vi "Auto.vi"() -> ()   [LabVIEW 2020]
uses:
  Global_Variable/A180648.vi
  Global_Variable/Global.vi
  Global_Variable/System_Conf.vi
  <userlib>/_MGI/1D Array/MGI Running Average/MGI Running Average(DBL).vi
  <userlib>/_MGI/1D Array/MGI Running Average/MGI Running Average(SGL).vi
  Libraries/S7/S7.lvlib
panel:
  out "磨合正向初始化":bool
  out "磨合逆向初始化":bool
  out "试验项_Event":refnum<user-event>
  out "产品变更_Event":refnum<user-event>
  out "NVH":bool=TRUE
  out "T1+T2":dbl
  out "T2":dbl
  out "T1":dbl
  out "吸收电流":sgl
  out "输出扭矩(大)":sgl
  out "输入扭矩":sgl
  out "力特性逆向去程":bool
  out "力特性正向去程":bool
  out "力特性逆向回程":bool
  out "力特性正向回程":bool
  out "逆向空载正向初始化":bool
  out "逆向空载逆向初始化":bool
  out "功能正向初始化":bool
  out "功能逆向初始化":bool
  out "空载逆向初始化":bool
  out "空载正向初始化":bool
  out "布尔":bool=TRUE
  out "当前车速":i32
  out "试验项目":T1(tab)
  out "空载试验":cluster{dbl[], dbl[]}[](graph)
  out "功能试验":cluster{dbl[], dbl[]}[](graph)
  out "力特性试验":cluster{dbl[], dbl[]}[](graph)
  out "电流特性试验":cluster{dbl[], dbl[]}[](graph)
  out "传感器特性试验":cluster{dbl[], dbl[]}[](graph)
  out "逆向空载试验":cluster{dbl[], dbl[]}[](graph)
  out "磨合":cluster{dbl[], dbl[]}[](graph)
  out "振动2NHV-FFT":cluster{"f0":dbl, "df":dbl, "magnitude":dbl[]}[](graph)
  out "振动1NVH-FFT":cluster{"f0":dbl, "df":dbl, "magnitude":dbl[]}[](graph)
  in  "判定结果":bool[][](array[boolean])=[[TRUE]]
  in  "STEP":string
  # "车速0"
  # "车速1"
  # "车速2"
  # "车速3"
  # "车速4"
  # "车速5"
  # "车速0"
  # "车速1"
  # "车速2"
  # "车速3"
  # "车速4"
  # "车速5"
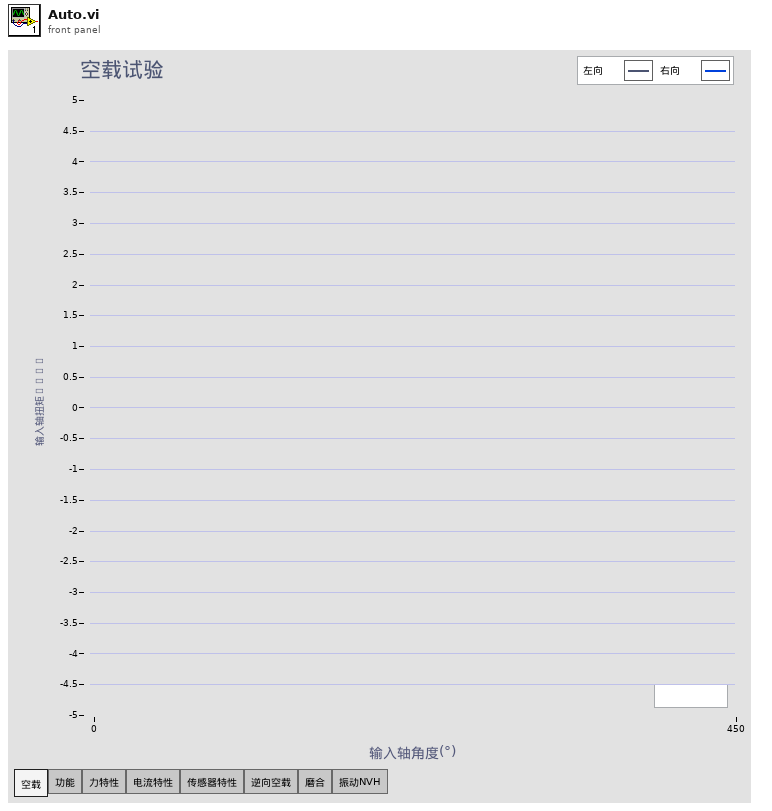
[diagram p1: front panel]
types:
  T1 = enum32{"空载", "功能", "力特性", "电流特性", "传感器特性", "逆向空载", "磨合", "振动NVH"}
  T2 = enum32{"Invalid", "Standard", "Closed", "Hidden", "Minimized", "Maximized"}
  T3 = enum32{"空载", "功能", "力特性", "电流特性", "传感器特性", "逆向空载", "振动NVH", "磨合", "完成"}
  T4 = enum16{"Left Button", "Center Button", "Right Button", "Window Close"}
  T5 = enum16{"角度标定状态", "角度标定", "角度标定清除", "扭矩标定状态", "扭矩标定", "扭矩标定清除", "内部软件版本号", "客户软件版本号"}
  T6 = enum16{"客户软件版本号", "角度标定状态", "角度标定", "角度标定清除", "扭矩标定状态", "扭矩标定", "扭矩标定清除", "内部软件版本号"}
  T7 = cluster{"输入轴扭矩":dbl, "输出轴扭矩小量程":dbl, "输出轴扭矩大量程":dbl}
  T8 = typedef "System_conf.ctl" = cluster{"空载滤波":bool, "逆向空载滤波":bool, "空载扭矩系数":dbl, "逆向空载扭矩系数":dbl}
  T9 = cluster{"扭矩判定范围":cluster{"单位":string, "下限":dbl, "上限":dbl}, "正向扭矩最大值":cluster{"单位":string, "下限":dbl, "上限":dbl}, "正向扭矩最小值":cluster{"单位":string, "下限":dbl, "上限":dbl}, "正向扭矩平均值":cluster{"单位":string, "下限":dbl, "上限":dbl}, "正向扭矩波动值":cluster{"单位":string, "下限":dbl, "上限":dbl}, "逆向扭矩最大值":cluster{"单位":string, "下限":dbl, "上限":dbl}, "逆向扭矩最小值":cluster{"单位":string, "下限":dbl, "上限":dbl}, "逆向扭矩平均值":cluster{"单位":string, "下限":dbl, "上限":dbl}, "逆向扭矩波动值":cluster{"单位":string, "下限":dbl, "上限":dbl}, "正逆向扭矩差值":cluster{"单位":string, "下限":dbl, "上限":dbl}, "启动力矩":cluster{"单位":string, "下限":dbl, "上限":dbl}}
  T10 = cluster{"扭矩判定范围":cluster{"单位":string, "下限":dbl, "上限":dbl}, "正向扭矩最大值":cluster{"单位":string, "下限":dbl, "上限":dbl}, "正向扭矩最小值":cluster{"单位":string, "下限":dbl, "上限":dbl}, "正向扭矩平均值":cluster{"单位":string, "下限":dbl, "上限":dbl}, "正向扭矩波动值":cluster{"单位":string, "下限":dbl, "上限":dbl}, "逆向扭矩最大值":cluster{"单位":string, "下限":dbl, "上限":dbl}, "逆向扭矩最小值":cluster{"单位":string, "下限":dbl, "上限":dbl}, "逆向扭矩平均值":cluster{"单位":string, "下限":dbl, "上限":dbl}, "逆向扭矩波动值":cluster{"单位":string, "下限":dbl, "上限":dbl}, "正逆向扭矩差值":cluster{"单位":string, "下限":dbl, "上限":dbl}}
  T11 = cluster{"对称性检测点":cluster{"单位":string, "下限":dbl, "上限":dbl}, "对称度":cluster{"单位":string, "下限":dbl, "上限":dbl}, "目标输出扭矩1":cluster{"单位":string, "下限":dbl, "上限":dbl}, "目标1正向输入扭矩":cluster{"单位":string, "下限":dbl, "上限":dbl}, "目标1逆向输入扭矩":cluster{"单位":string, "下限":dbl, "上限":dbl}, "目标1正逆向扭矩差":cluster{"单位":string, "下限":dbl, "上限":dbl}, "目标1输入扭矩滞后":cluster{"单位":string, "下限":dbl, "上限":dbl}, "目标输出扭矩2":cluster{"单位":string, "下限":dbl, "上限":dbl}, "目标2正向输入扭矩":cluster{"单位":string, "下限":dbl, "上限":dbl}, "目标2逆向输入扭矩":cluster{"单位":string, "下限":dbl, "上限":dbl}, "目标2正逆向扭矩差":cluster{"单位":string, "下限":dbl, "上限":dbl}, "目标2输入扭矩滞后":cluster{"单位":string, "下限":dbl, "上限":dbl}, "目标输出扭矩3":cluster{"单位":string, "下限":dbl, "上限":dbl}, "目标3正向输入扭矩":cluster{"单位":string, "下限":dbl, "上限":dbl}, "目标3逆向输入扭矩":cluster{"单位":string, "下限":dbl, "上限":dbl}, "目标3正逆向扭矩差":cluster{"单位":string, "下限":dbl, "上限":dbl}, "目标3输入扭矩滞后":cluster{"单位":string, "下限":dbl, "上限":dbl}, "目标输出扭矩4":cluster{"单位":string, "下限":dbl, "上限":dbl}, "目标4正向输入扭矩":cluster{"单位":string, "下限":dbl, "上限":dbl}, "目标4逆向输入扭矩":cluster{"单位":string, "下限":dbl, "上限":dbl}, "目标4正逆向扭矩差":cluster{"单位":string, "下限":dbl, "上限":dbl}, "目标4输入扭矩滞后":cluster{"单位":string, "下限":dbl, "上限":dbl}, "目标输出扭矩5":cluster{"单位":string, "下限":dbl, "上限":dbl}, "目标5正向输入扭矩":cluster{"单位":string, "下限":dbl, "上限":dbl}, "目标5逆向输入扭矩":cluster{"单位":string, "下限":dbl, "上限":dbl}, "目标5正逆向扭矩差":cluster{"单位":string, "下限":dbl, "上限":dbl}, "目标5输入扭矩滞后":cluster{"单位":string, "下限":dbl, "上限":dbl}}[]
  T12 = cluster{"主副信号和MAX":cluster{"单位":string, "下限":dbl, "上限":dbl}, "主副信号和MIN":cluster{"单位":string, "下限":dbl, "上限":dbl}, "主信号线性误差":cluster{"单位":string, "下限":dbl, "上限":dbl}, "副信号线性误差":cluster{"单位":string, "下限":dbl, "上限":dbl}, "主信号MAX":cluster{"单位":string, "下限":dbl, "上限":dbl}, "主信号MIN":cluster{"单位":string, "下限":dbl, "上限":dbl}, "副信号MAX":cluster{"单位":string, "下限":dbl, "上限":dbl}, "副信号MIN":cluster{"单位":string, "下限":dbl, "上限":dbl}, "中心偏移量":cluster{"单位":string, "下限":dbl, "上限":dbl}, "定点设置":cluster{"单位":string, "下限":dbl, "上限":dbl}, "定点左侧主信号":cluster{"单位":string, "下限":dbl, "上限":dbl}, "定点左侧副信号":cluster{"单位":string, "下限":dbl, "上限":dbl}, "定点右侧主信号":cluster{"单位":string, "下限":dbl, "上限":dbl}, "定点右侧副信号":cluster{"单位":string, "下限":dbl, "上限":dbl}}
  T13 = cluster{"对称性检测点":cluster{"单位":string, "下限":dbl, "上限":dbl}, "对称度":cluster{"单位":string, "下限":dbl, "上限":dbl}, "最大电流":cluster{"单位":string, "下限":dbl, "上限":dbl}, "目标输出电流1":cluster{"单位":string, "下限":dbl, "上限":dbl}, "目标1正向输入扭矩":cluster{"单位":string, "下限":dbl, "上限":dbl}, "目标1逆向输入扭矩":cluster{"单位":string, "下限":dbl, "上限":dbl}, "目标1正逆向扭矩差":cluster{"单位":string, "下限":dbl, "上限":dbl}, "目标1输入扭矩滞后":cluster{"单位":string, "下限":dbl, "上限":dbl}, "目标输出电流2":cluster{"单位":string, "下限":dbl, "上限":dbl}, "目标2正向输入扭矩":cluster{"单位":string, "下限":dbl, "上限":dbl}, "目标2逆向输入扭矩":cluster{"单位":string, "下限":dbl, "上限":dbl}, "目标2正逆向扭矩差":cluster{"单位":string, "下限":dbl, "上限":dbl}, "目标2输入扭矩滞后":cluster{"单位":string, "下限":dbl, "上限":dbl}, "目标输出电流3":cluster{"单位":string, "下限":dbl, "上限":dbl}, "目标3正向输入扭矩":cluster{"单位":string, "下限":dbl, "上限":dbl}, "目标3逆向输入扭矩":cluster{"单位":string, "下限":dbl, "上限":dbl}, "目标3正逆向扭矩差":cluster{"单位":string, "下限":dbl, "上限":dbl}, "目标3输入扭矩滞后":cluster{"单位":string, "下限":dbl, "上限":dbl}, "目标输出电流4":cluster{"单位":string, "下限":dbl, "上限":dbl}, "目标4正向输入扭矩":cluster{"单位":string, "下限":dbl, "上限":dbl}, "目标4逆向输入扭矩":cluster{"单位":string, "下限":dbl, "上限":dbl}, "目标4正逆向扭矩差":cluster{"单位":string, "下限":dbl, "上限":dbl}, "目标4输入扭矩滞后":cluster{"单位":string, "下限":dbl, "上限":dbl}, "目标输出电流5":cluster{"单位":string, "下限":dbl, "上限":dbl}, "目标5正向输入扭矩":cluster{"单位":string, "下限":dbl, "上限":dbl}, "目标5逆向输入扭矩":cluster{"单位":string, "下限":dbl, "上限":dbl}, "目标5正逆向扭矩差":cluster{"单位":string, "下限":dbl, "上限":dbl}, "目标5输入扭矩滞后":cluster{"单位":string, "下限":dbl, "上限":dbl}}[]
  T14 = cluster{"振动1频率检测段1范围":cluster{"单位":string, "下限":dbl, "上限":dbl}, "振动1频率检测段2范围":cluster{"单位":string, "下限":dbl, "上限":dbl}, "振动1频率检测段3范围":cluster{"单位":string, "下限":dbl, "上限":dbl}, "振动1频率检测段4范围":cluster{"单位":string, "下限":dbl, "上限":dbl}, "振动1频率检测段5范围":cluster{"单位":string, "下限":dbl, "上限":dbl}, "振动2频率检测段1范围":cluster{"单位":string, "下限":dbl, "上限":dbl}, "振动2频率检测段2范围":cluster{"单位":string, "下限":dbl, "上限":dbl}, "振动2频率检测段3范围":cluster{"单位":string, "下限":dbl, "上限":dbl}, "振动2频率检测段4范围":cluster{"单位":string, "下限":dbl, "上限":dbl}, "振动2频率检测段5范围":cluster{"单位":string, "下限":dbl, "上限":dbl}}
  T15 = cluster{"振动1频率检测段1振幅":cluster{"单位":string, "下限":dbl, "上限":dbl}, "振动1频率检测段2振幅":cluster{"单位":string, "下限":dbl, "上限":dbl}, "振动1频率检测段3振幅":cluster{"单位":string, "下限":dbl, "上限":dbl}, "振动1频率检测段4振幅":cluster{"单位":string, "下限":dbl, "上限":dbl}, "振动1频率检测段5振幅":cluster{"单位":string, "下限":dbl, "上限":dbl}, "振动2频率检测段1振幅":cluster{"单位":string, "下限":dbl, "上限":dbl}, "振动2频率检测段2振幅":cluster{"单位":string, "下限":dbl, "上限":dbl}, "振动2频率检测段3振幅":cluster{"单位":string, "下限":dbl, "上限":dbl}, "振动2频率检测段4振幅":cluster{"单位":string, "下限":dbl, "上限":dbl}, "振动2频率检测段5振幅":cluster{"单位":string, "下限":dbl, "上限":dbl}}
  T16 = cluster{"扭矩判定范围":cluster{"单位":string, "下限":dbl, "上限":dbl}, "正向扭矩最大值":cluster{"单位":string, "下限":dbl, "上限":dbl}, "正向扭矩最小值":cluster{"单位":string, "下限":dbl, "上限":dbl}, "正向扭矩平均值":cluster{"单位":string, "下限":dbl, "上限":dbl}, "正向扭矩波动值":cluster{"单位":string, "下限":dbl, "上限":dbl}, "逆向扭矩最大值":cluster{"单位":string, "下限":dbl, "上限":dbl}, "逆向扭矩最小值":cluster{"单位":string, "下限":dbl, "上限":dbl}, "逆向扭矩平均值":cluster{"单位":string, "下限":dbl, "上限":dbl}, "逆向扭矩波动值":cluster{"单位":string, "下限":dbl, "上限":dbl}, "正逆向扭矩差值":cluster{"单位":string, "下限":dbl, "上限":dbl}, "启动扭矩范围":cluster{"单位":string, "下限":dbl, "上限":dbl}, "启动扭矩":cluster{"单位":string, "下限":dbl, "上限":dbl}}
  T17 = cluster{"试验速度":dbl, "试验角度":dbl, "负载扭矩":dbl, "保护扭矩":dbl}
  T18 = cluster{"输入旋转位移":sgl, "输入移载位移":sgl, "工装移载位移":sgl, "输入编码位移":sgl, "输入扭矩":sgl, "输出扭矩(小)":sgl, "输出扭矩(大)":sgl, "吸收电流":sgl}
  T19 = typedef "svc_Spectrum Info.ctl" = cluster{"channel name":string, "description":string, "x-axis units":T20, "spectral info":cluster{"spectrum type":T21, "linear/dB":enum16{"linear", "dB"}, "window":u16, "window size":i32, "FFT size":i32}, "engineering units":T22, "custom label":string, "dB reference [EU]":dbl, "peak units":enum16{"rms", "peak", "peak-peak"}, "weighting filter":T23, "spectral density?":bool, "unit label":string, "spectrum skewed?":bool, "complimentary spectrum units":T24}
  T20 = typedef "svc_X-Axis Units.ctl" = u16
  T21 = typedef "svc_Spectrum Type.ctl" = enum16{"FFT Spectrum [complex]", "Amplitude [Magnitude]", "Power [Magnitude^2]", "Cross Spectrum [complex]", "Frequency Response [Complex]"}
  T22 = typedef "svc_Engineering Units Text Ring.ctl" = u16
  T23 = typedef "svc_Weighting Filter Text Ring.ctl" = u16
  T24 = typedef "svc_Complimentary Spectrum Units.ctl" = enum16{"none", "radians", "degrees", "cycles", "imaginary"}
  T25 = cluster{"启用助力":dbl, "试验速度":dbl, "试验角度":dbl, "保护扭矩":dbl}
  T26 = typedef "lveventtype.ctl" = enum32{"Null", "Timeout", "Annotation Menu Selection", "Annotation Menu Selection?", "App Instance Close", "App Instance Close?", "Autoscale Range Change", "Bookmark Info Change", "Cell Edit", "Cell Edit?", "Cursor Grab", "Cursor Grab?", "Cursor Menu Selection", "Cursor Menu Selection?", "Cursor Move", "Cursor Release", "Data Change", "Direction Change", "Display State Change", "Drag Ended", "Drag Enter", "Drag Leave", "Drag Over", "Drag Source Update", "Drag Starting", "Drag Starting?", "Drop", "Exec State Change", "Key Down", "Key Down?", "Key Repeat", "Key Repeat?", "Key Up", "Listbox Double Click", "Menu Activation?", "Menu Selection (App)", "Menu Selection? (App)", "Menu Selection (User)", "Mouse Down", "Mouse Down?", "Mouse Enter", "Mouse Leave", "Mouse Move", "Mouse Up", "Mouse Wheel", "NI Security User Change (App)", "Pane Size", "Panel Close", "Panel Close?", "Panel Resize", "Plot Attribute Change", "Scale Range Change", "Shortcut Menu Activation?", "Shortcut Menu Selection (App)", "Shortcut Menu Selection? (App)", "Shortcut Menu Selection (User)", "Tree Double Click", "Tree Drag", "Tree Drag?", "Tree Drop", "Tree Drop?", "Tree Item Close", "Tree Item Close?", "Tree Item Open", "Tree Item Open?", "User Event", "Value Change"}
  T27 = typedef "LVPoint32TypeDef.ctl" = cluster{"Horizontal":i32, "Vertical":i32}
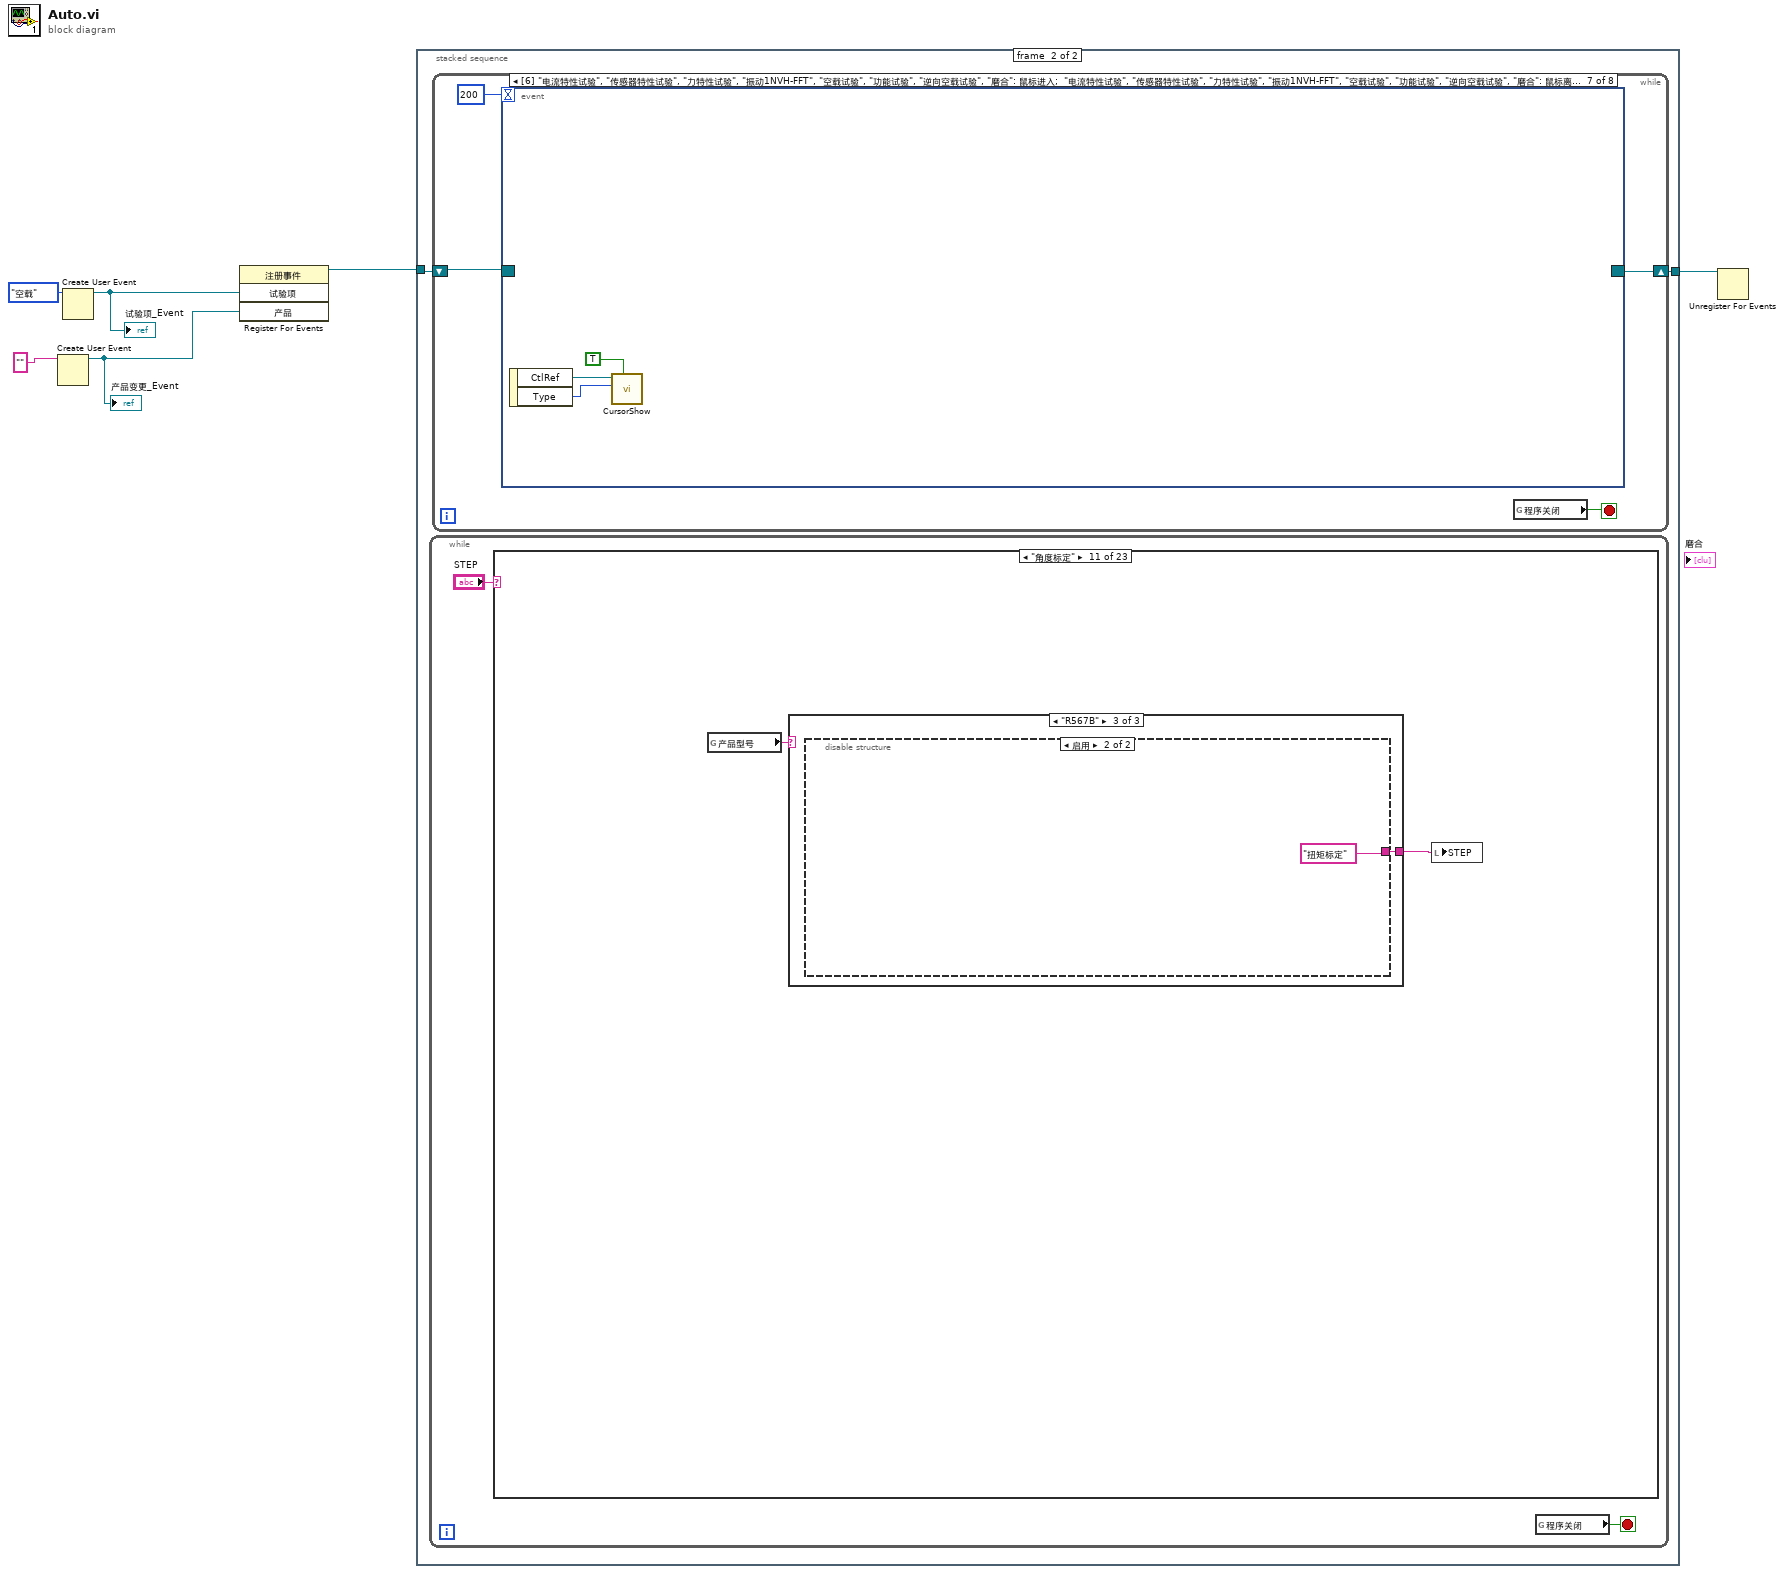
[diagram p0: block diagram]
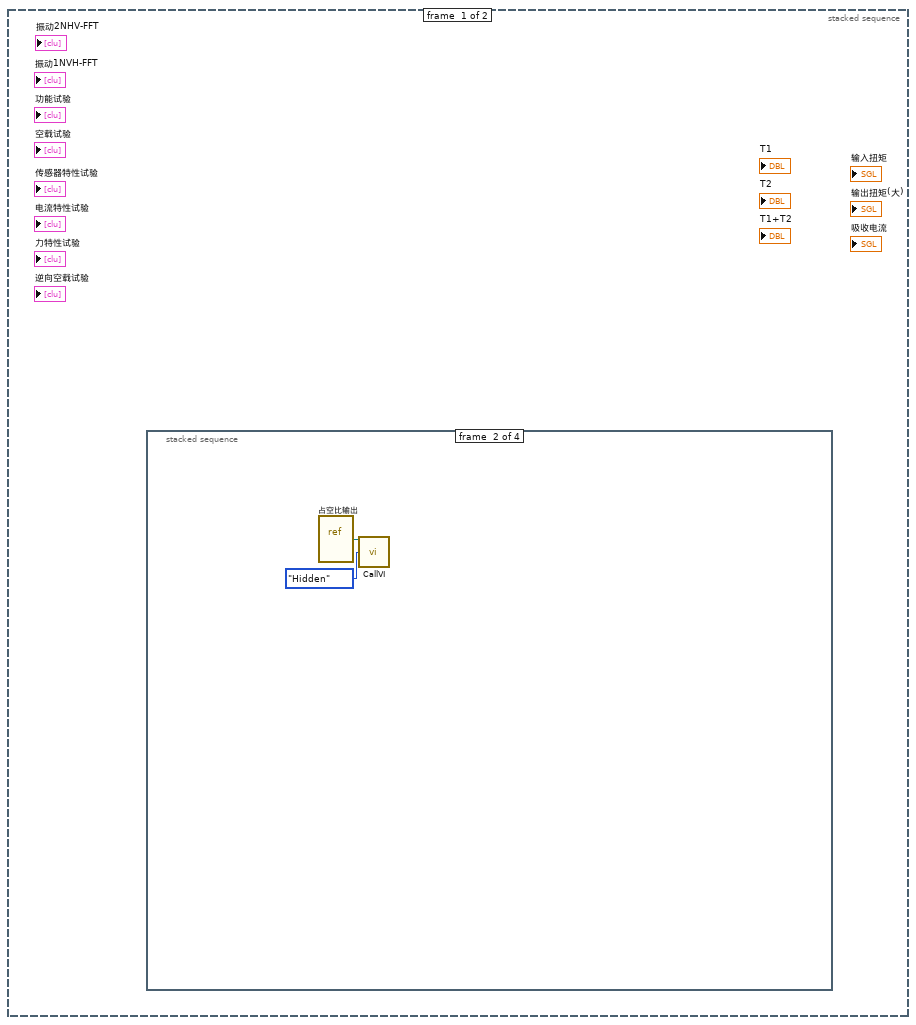
[diagram p2: hidden frame]
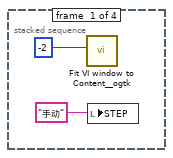
[diagram p3: hidden frame]
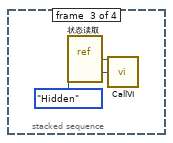
[diagram p4: hidden frame]
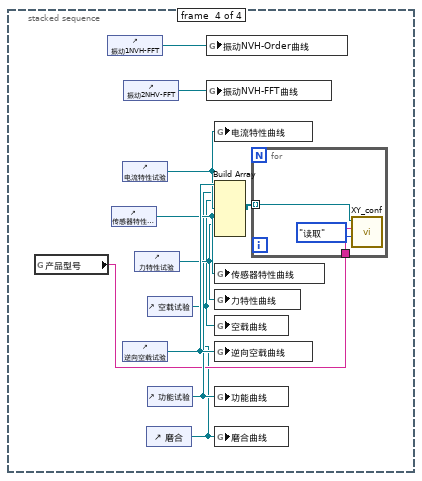
[diagram p5: hidden frame]
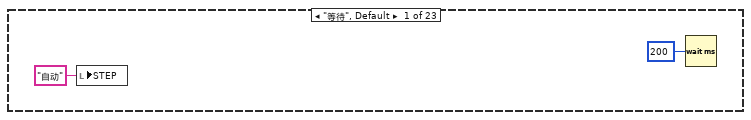
[diagram p6: hidden frame]
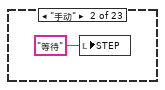
[diagram p7: hidden frame]
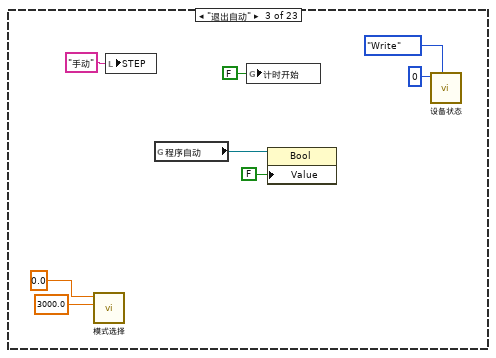
[diagram p8: hidden frame]
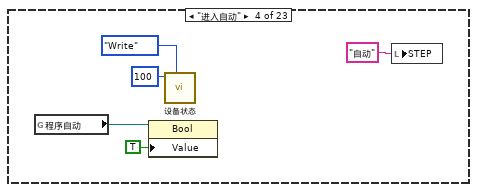
[diagram p9: hidden frame]
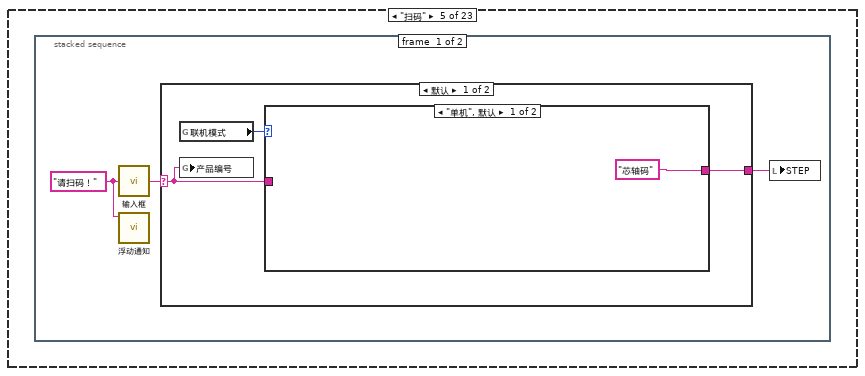
[diagram p10: hidden frame]
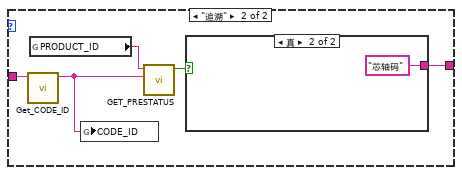
[diagram p11: hidden frame]
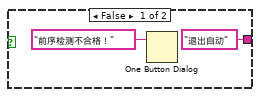
[diagram p12: hidden frame]
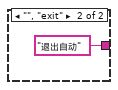
[diagram p13: hidden frame]
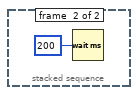
[diagram p14: hidden frame]
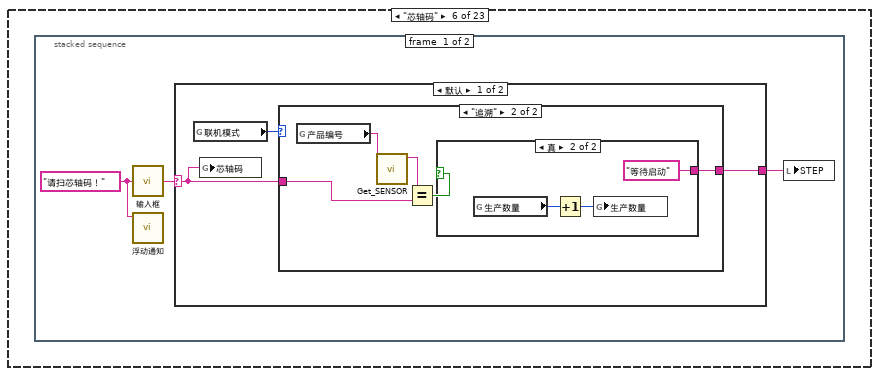
[diagram p15: hidden frame]
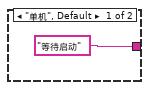
[diagram p16: hidden frame]
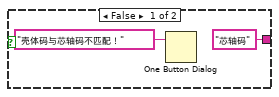
[diagram p17: hidden frame]
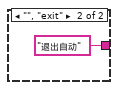
[diagram p18: hidden frame]
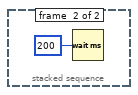
[diagram p19: hidden frame]
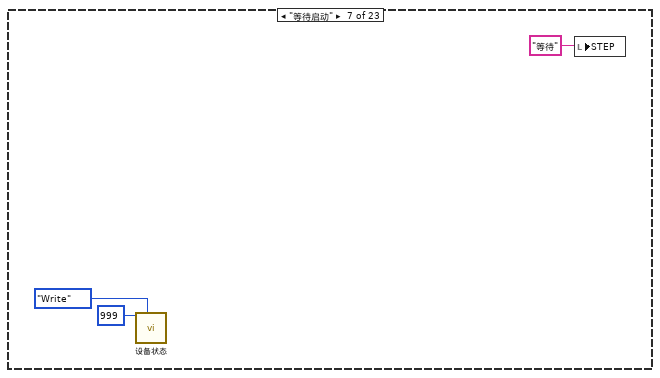
[diagram p20: hidden frame]
diagram:
  n1 = Create User Event(user event datatype="" ("产品")) -> (user event=w1:refnum<user-event>)  [unwired: 1 in, 1 out]
  "产品变更_Event" <- w1
  n2 = Create User Event(user event datatype=T1."空载" ("试验项")) -> (user event=w4:refnum<user-event>)  [unwired: 1 in, 1 out]
  "试验项_Event" <- w4
  n3 = register-events(w4, w1) -> (reference out=w5:refnum<event-registration>)  [unwired: 2 in, 1 out]
  n4 = stacked-sequence {
    tunnel: w5 -> [_ w28]
    tunnel: [_ w27] -> w3
    frame #0 {
      n5 = stacked-sequence {
        frame #0 {
          n6 = call <userlib>:"Fit VI window to Content__ogtk.vi"("border spacing (2 px)"=-2) -> ()  [unwired: 5 in, 2 out]
          n7 = local write "STEP"("手动" ("STEP")) -> ()
        }
        frame #1 {
          n8 = vi-ref "占空比输出.vi"() -> (w10:refnum<vi>)
          n9 = call "CallVI.vi"("VI引用"=w10, "状态"=T2."Hidden") -> ()  [unwired: 12 in, 2 out]
        }
        frame #2 {
          n10 = vi-ref "状态读取.vi"() -> (w12:refnum<vi>)
          n11 = call "CallVI.vi"("VI引用"=w12, "状态"=T2."Hidden") -> ()  [unwired: 12 in, 2 out]
        }
        frame #3 {
          n12 = global read "Global.vi" "产品型号"() -> (w14:string)
          n13 = control-ref of="振动1NVH-FFT"() -> (w22:refnum<vi>)
          n14 = control-ref of="传感器特性试验"() -> (w19:refnum<vi>)
          n15 = control-ref of="电流特性试验"() -> (w20:refnum<vi>)
          n16 = control-ref of="逆向空载试验"() -> (w21:refnum<vi>)
          n17 = control-ref of="振动2NHV-FFT"() -> (w23:refnum<vi>)
          n18 = control-ref of="力特性试验"() -> (w18:refnum<vi>)
          n19 = control-ref of="磨合"() -> (w13:refnum<vi>)
          n20 = control-ref of="空载试验"() -> (w16:refnum<vi>)
          n21 = control-ref of="功能试验"() -> (w17:refnum<vi>)
          n22 = global write "A180648.vi" "振动NVH-Order曲线"(w22) -> ()
          n23 = global write "A180648.vi" "振动NVH-FFT曲线"(w23) -> ()
          n24 = global write "A180648.vi" "电流特性曲线"(w20) -> ()
          n25 = Build Array(w21, w17, w16, w20, w19, w18, w13) -> (w15:refnum<vi>[])
          n26 = global write "A180648.vi" "传感器特性曲线"(w19) -> ()
          n27 = global write "A180648.vi" "力特性曲线"(w18) -> ()
          n28 = global write "A180648.vi" "空载曲线"(w16) -> ()
          n29 = global write "A180648.vi" "逆向空载曲线"(w21) -> ()
          n30 = global write "A180648.vi" "功能曲线"(w17) -> ()
          n31 = global write "A180648.vi" "磨合曲线"(w13) -> ()
          n32 = for {
            tunnel: w15 -> [w25] mode=indexing
            tunnel: w14 -> [w24]
            n33 = call "XY_conf.vi"("方式"=enum16{"写入", "读取"}."读取", "产品"=w24, "XY图引用"=w25) -> ()  [unwired: 4 in, 1 out]
          }
        }
      }
    }
    frame #1 {
      n34 = while {
        stop <- w30 stop-if-true
        n35 = case shown="\"角度标定\"" "STEP" {
          frame "等待", Default {
            n36 = local write "STEP"("自动" ("STEP")) -> ()
            n37 = Wait (ms)(milliseconds to wait=u32 200 ("等待时间（毫秒）")) -> ()  [unwired: 1 out]
          }
          frame "手动" {
            n38 = local write "STEP"("等待" ("STEP")) -> ()
          }
          frame "退出自动" {
            n39 = call-poly "模式选择.vi"("Max Torque"=sgl 3000.0, "Velocity"=sgl 0.0) -> ()  [unwired: 9 in, 1 out]
            n40 = local write "STEP"("手动" ("STEP")) -> ()
            n41 = global read "Global.vi" "程序自动"() -> (w37:refnum<vi>)
            n42 = global write "Global.vi" "计时开始"(FALSE ("计时开始")) -> ()
            n43 = property class="Bool"(reference=w37, "Value"=FALSE) -> ()  [unwired: 1 in, 2 out]
            n44 = call "设备状态.vi"("枚举"=enum16{"Read", "Write"}."Write", "Status_Write"=i16 0) -> ()  [unwired: 9 in, 1 out]
          }
          frame "进入自动" {
            n45 = global read "Global.vi" "程序自动"() -> (w43:refnum<vi>)
            n46 = property class="Bool"(reference=w43, "Value"=TRUE) -> ()  [unwired: 1 in, 2 out]
            n47 = call "设备状态.vi"("枚举"=enum16{"Read", "Write"}."Write", "Status_Write"=i16 100) -> ()  [unwired: 9 in, 1 out]
            n48 = local write "STEP"("自动" ("STEP")) -> ()
          }
          frame "扫码" {
            n49 = stacked-sequence {
              frame #0 {
                w48 = "请扫码！" ("提示信息")
                n50 = call "输入框.vi"("提示信息"=w48) -> ("条形码输出"=w49:string)
                n51 = call "浮动通知.vi"("通知内容"=w48) -> ()  [unwired: 11 in]
                n52 = case shown="默认" w49 {
                  selector: w49 -> [w51 _]
                  tunnel: [w52 "退出自动" ("State(s) in Front (\"\")")] -> w47
                  frame Default {
                    n53 = global read "Global.vi" "联机模式"() -> (w50:enum16{"单机", "追溯"})
                    n54 = global write "Global.vi" "产品编号"(w51) -> ()
                    n55 = case shown="\"单机\", 默认" w50 {
                      tunnel: ["芯轴码" ("State(s) in Front (\"\")") w58] -> w52
                      tunnel: w51 -> [_ w55]
                      frame "单机", Default {
                      }
                      frame "追溯" {
                        n56 = call "Get_CODE_ID.vi"("CODE_MAIN"=w55) -> ("CODE_ID"=w54:string)  [unwired: 10 in]
                        n57 = global read "追溯Global.vi" "PRODUCT_ID"() -> (w57:string)
                        n58 = global write "追溯Global.vi" "CODE_ID"(w54) -> ()
                        n59 = call "GET_PRESTATUS.vi"("CODE_ID"=w54, "PRODUCT_ID"=w57) -> ("OK?"=w56:bool)  [unwired: 9 in]
                        n60 = case shown="真" w56 {
                          tunnel: ["退出自动" ("State(s) in Front (\"\")") "芯轴码" ("State(s) in Front (\"\")")] -> w58
                          frame False {
                            n61 = One Button Dialog(message="前序检测不合格！" ("消息")) -> ()  [unwired: 1 in, 1 out]
                          }
                          frame True {
                          }
                        }
                      }
                    }
                  }
                  frame "", "exit" {
                  }
                }
                n62 = local write "STEP"(w47) -> ()
              }
              frame #1 {
                n63 = Wait (ms)(milliseconds to wait=u32 200 ("等待时间（毫秒）")) -> ()  [unwired: 1 out]
              }
            }
          }
          frame "芯轴码" {
            n64 = stacked-sequence {
              frame #0 {
                w65 = "请扫芯轴码！" ("提示信息")
                n65 = call "输入框.vi"("提示信息"=w65) -> ("条形码输出"=w66:string)
                n66 = call "浮动通知.vi"("通知内容"=w65) -> ()  [unwired: 11 in]
                n67 = case shown="默认" w66 {
                  selector: w66 -> [w68 _]
                  tunnel: [w69 "退出自动" ("State(s) in Front (\"\")")] -> w64
                  frame Default {
                    n68 = global read "Global.vi" "联机模式"() -> (w67:enum16{"单机", "追溯"})
                    n69 = global write "Global.vi" "芯轴码"(w68) -> ()
                    n70 = case shown="\"追溯\"" w67 {
                      tunnel: ["等待启动" ("State(s) in Front (\"\")") w75] -> w69
                      tunnel: w68 -> [_ w72]
                      frame "单机", Default {
                      }
                      frame "追溯" {
                        n71 = global read "Global.vi" "产品编号"() -> (w74:string)
                        n72 = call "Get_SENSOR.vi"("CODE_MAIN"=w74) -> ("CODE_SENSOR"=w73:string)  [unwired: 10 in]
                        n73 = Equal?(x=w73, y=w72) -> (x = y?=w71:bool)
                        n74 = case shown="真" w71 {
                          tunnel: ["芯轴码" ("State(s) in Front (\"\")") "等待启动" ("State(s) in Front (\"\")")] -> w75
                          frame False {
                            n75 = One Button Dialog(message="壳体码与芯轴码不匹配！" ("消息")) -> ()  [unwired: 1 in, 1 out]
                          }
                          frame True {
                            n76 = global read "Global.vi" "生产数量"() -> (w78:i32)
                            n77 = Increment(x=w78) -> (x+1=w79:i32)
                            n78 = global write "Global.vi" "生产数量"(w79) -> ()
                          }
                        }
                      }
                    }
                  }
                  frame "", "exit" {
                  }
                }
                n79 = local write "STEP"(w64) -> ()
              }
              frame #1 {
                n80 = Wait (ms)(milliseconds to wait=u32 200 ("等待时间（毫秒）")) -> ()  [unwired: 1 out]
              }
            }
          }
          frame "等待启动" {
            n81 = call "设备状态.vi"("枚举"=enum16{"Read", "Write"}."Write", "Status_Write"=i16 999 ("设备状态")) -> ()  [unwired: 9 in, 1 out]
            n82 = local write "STEP"("等待" ("STEP")) -> ()
          }
          frame "初始化" {
            n83 = stacked-sequence {
              frame #0 {
                n84 = global write "Global.vi" "IO_Stop"(TRUE ("IO_Stop")) -> ()
                n85 = global write "Global.vi" "计时开始"(TRUE ("计时开始")) -> ()
                n86 = local write "判定结果"(bool[][] [] ("判定结果")) -> ()
                n87 = global write "A180648.vi" "当前车速"(u16 0 ("当前车速")) -> ()
                n88 = global read "Global.vi" "产品型号"() -> (w86:string)
                n89 = call "Demarcate.vi"("Mode"=enum16{"Read", "Write"}."Read", "Section"=w86) -> ("Sensor OUT"=w90:T7)  [unwired: 8 in, 1 out]
                n90 = call "Demarcate2.vi"("Mode"=enum16{"Read", "Write"}."Read", "Section"=w86) -> ("Sensor OUT"=w89:T7)  [unwired: 8 in, 1 out]
                n91 = call "System_Conf_RW.vi"("Mode"=enum16{"Read", "Write"}."Read", "Section"=w86) -> ("system_out"=w93:T8)  [unwired: 8 in, 1 out]
                n92 = global write "传感器偏移.vi" "传感器偏移"(w90) -> ()
                n93 = global write "传感器偏移.vi" "传感器手动修正"(w89) -> ()
                n94 = global write "System_Conf.vi" "system"(w93) -> ()
                "当前车速" <- 0 ("当前车速")
              }
              frame #1 {
                w98 = TRUE
                "逆向空载正向初始化" <- w98
                "逆向空载逆向初始化" <- w98
                "空载正向初始化" <- w98
                "空载逆向初始化" <- w98
                "功能正向初始化" <- w98
                "功能逆向初始化" <- w98
                "力特性逆向去程" <- w98
                "力特性正向去程" <- w98
                "力特性逆向回程" <- w98
                "力特性正向回程" <- w98
                "磨合正向初始化" <- w98
                "磨合逆向初始化" <- w98
              }
              frame #2 {
                n95 = for {
                  N: 24 -> [_]
                  tunnel: [cluster{dbl[], dbl[]} {[], []}] -> w99 mode=indexing
                  tunnel: [cluster{"f0":dbl, "df":dbl, "magnitude":dbl[]} {"f0"=0.0, "df"=0.0, "magnitude"=[]} ("power spectrum [dB EU]")] -> w100 mode=indexing
                }
                n96 = local write "传感器特性试验"(w99) -> ()
                n97 = local write "逆向空载试验"(w99) -> ()
                n98 = local write "力特性试验"(w99) -> ()
                n99 = local write "电流特性试验"(w99) -> ()
                n100 = local write "空载试验"(w99) -> ()
                n101 = local write "功能试验"(w99) -> ()
                n102 = local write "磨合"(w99) -> ()
                n103 = local write "振动2NHV-FFT"(w100) -> ()
                n104 = local write "振动1NVH-FFT"(w100) -> ()
              }
              frame #3 {
                n105 = global read "Global.vi" "Result"() -> (w106:refnum<vi>)
                n106 = property class="Tbl"(reference=w106, "Value"=string[][] []) -> (reference out=w107:refnum<vi>, error out=w108:errorcluster)  [unwired: 1 in]
                n107 = property class="Tbl"(reference=w107, error in=w108, "Row Headers[]"=string[] [] ("列首字符串[]")) -> ()  [unwired: 2 out]
              }
              frame #4 {
                n108 = global read "A180648.vi" "LED-传感器特性"() -> (w114:refnum<vi>)
                n109 = global read "A180648.vi" "LED-振动NVH"() -> (w110:refnum<vi>)
                n110 = global read "A180648.vi" "LED-电流特性"() -> (w115:refnum<vi>)
                n111 = global read "A180648.vi" "LED-逆向空载"() -> (w111:refnum<vi>)
                n112 = global read "A180648.vi" "LED-磨合"() -> (w109:refnum<vi>)
                n113 = global read "A180648.vi" "LED-力特性"() -> (w112:refnum<vi>)
                n114 = global read "A180648.vi" "LED-功能"() -> (w117:refnum<vi>)
                n115 = global read "A180648.vi" "LED-空载"() -> (w113:refnum<vi>)
                n116 = Build Array(w114, w115, w117, w113, w112, w111, w110, w109) -> (w116:refnum<vi>[])
                n117 = for {
                  tunnel: w116 -> [w118] mode=indexing
                  n118 = property class="Bool"(reference=w118, "Colors [4]"=cluster{u32, u32}[] [{12369084, 12369084}] ("颜色[4]")) -> ()  [unwired: 1 in, 2 out]
                }
              }
              frame #5 {
                w123 = 1 ("维数大小")
                n119 = Initialize Array(" " ("字符串"), w123, w123, w123) -> (w125:string[][][])
                n120 = global write "Global.vi" "STOP_NVH"(FALSE ("STOP_NVH")) -> ()
                n121 = global write "A180648.vi" "当前检测项"(T3."空载" ("当前检测项")) -> ()
                n122 = global write "A180648.vi" "检测结果"(w125) -> ()
                n123 = global write "Global.vi" "重试次数"(0 ("重试次数")) -> ()
              }
              frame #6 {
                n124 = global read "Global.vi" "启用CAN"() -> (w129:bool)
                n125 = Select(t="CAN初始化" ("STEP"), s=w129, f="K-Line初始化" ("STEP")) -> (s? t:f=w126:string)
                n126 = local write "STEP"(w126) -> ()
              }
            }
          }
          frame "CAN初始化" {
            n127 = while {
              tunnel: [w134] -> w130
              stop <- w135 stop-if-true
              n128 = global read "Global.vi" "CAN软件版本号"() -> (w132:string)
              n129 = call "Can软件版本号.vi"() -> ("软件版本号"=w133:string)  [unwired: 11 in]
              n130 = Equal?(x=w133, y=w132) -> (x = y?=w136:bool)
              n131 = global write "Global.vi" "软件版本号"(w133) -> ()
              n132 = case shown="假" w136 {
                tunnel: [w145 T4."Center Button" ("Which Button?")] -> w131
                tunnel: w133 -> [w148 _]
                tunnel: w132 -> [w147 _]
                frame False {
                  n133 = global read "Global.vi" "重试次数"() -> (w146:i32)
                  n134 = Increment(x=w146) -> (x+1=w143:i32)
                  n135 = Greater?(x=w143, y=1) -> (0:w144:bool)
                  n136 = global write "Global.vi" "重试次数"(w143) -> ()
                  n137 = case shown="假" w144 {
                    tunnel: w148 -> [_ w158]
                    tunnel: w147 -> [_ w157]
                    tunnel: [T4."Left Button" ("Which Button?") w150] -> w145
                    frame False {
                    }
                    frame True {
                      n138 = Format Into String(format string="软件版本号不匹配！\nECU软件版本号：%s\n预期软件版本号：%s" ("message"), w158, w157) -> (resulting string=w151:string)  [unwired: 2 in, 1 out]
                      n139 = call <vilib>:"Three Button Dialog.vi"("Allow user to close window? (TRUE)"=FALSE, "Right Button Text (\"Cancel\")"="取消" ("Right Button Text (\"Cancel\")"), "Center Button Text (\"No\")"="忽略" ("Center Button Text (\"No\")"), "Left Button Text (\"Yes\")"="重试" ("Left Button Text (\"Yes\")"), "message"=w151) -> ("Which Button?"=w150:T4)  [unwired: 6 in]
                    }
                  }
                }
                frame True {
                }
              }
              n140 = case shown="\"Center Button\"" w131 {
                tunnel: [FALSE TRUE TRUE] -> w135
                tunnel: [_ "角度标定" "退出自动"] -> w134
                frame "Left Button", Default {
                }
                frame "Center Button" {
                }
                frame "Right Button" {
                }
              }
            }
            n141 = local write "STEP"(w130) -> ()
          }
          frame "K-Line初始化" {
            n142 = global read "Global.vi" "启用K-line诊断"() -> (w160:bool)
            n143 = case shown="真" w160 {
              frame False {
                n144 = local write "STEP"("试验项" ("STEP")) -> ()
              }
              frame True {
                n145 = global read "Global.vi" "VISA resource name"() -> (w166:refnum<visa-resource-name>)
                n146 = global read "Global.vi" "K-Line波特率"() -> (w165:u32)
                n147 = global read "Global.vi" "诊断指令"() -> (w164:string[][])
                n148 = call "K线诊断.vi"("K线诊断"=w164, "波特率"=w165, "VISA resource name"=w166) -> ("字符串"=w162:string, "逻辑与"=w163:bool)  [unwired: 7 in]
                n149 = case shown="假" w163 {
                  tunnel: w162 -> [w173 _]
                  frame False {
                    n150 = global write "Global.vi" "K-Line状态"("NG" ("K-Line状态")) -> ()
                    n151 = call <vilib>:"Three Button Dialog.vi"("Allow user to close window? (TRUE)"=FALSE, "Window Title (\"\")"="K-Line诊断异常！" ("Window Title (\"\")"), "Right Button Text (\"Cancel\")"="中止" ("Right Button Text (\"Cancel\")"), "Center Button Text (\"No\")"="忽略" ("Center Button Text (\"No\")"), "Left Button Text (\"Yes\")"="重试" ("Left Button Text (\"Yes\")"), "message"=w173) -> ("Which Button?"=w167:T4)  [unwired: 5 in]
                    n152 = case shown="\"Center Button\"" w167 {
                      frame "Left Button", Default {
                        n153 = local write "STEP"("K-Line初始化" ("STEP")) -> ()
                      }
                      frame "Center Button" {
                        n154 = local write "STEP"("试验项" ("STEP")) -> ()
                      }
                      frame "Right Button" {
                        n155 = local write "STEP"("退出自动" ("STEP")) -> ()
                      }
                    }
                  }
                  frame True {
                    n156 = global write "Global.vi" "K-Line状态"("OK" ("K-Line状态")) -> ()
                    n157 = local write "STEP"("试验项" ("STEP")) -> ()
                    n158 = call "浮动通知.vi"("通知内容"="K-Line诊断正常！" ("Status")) -> ()  [unwired: 11 in]
                  }
                }
              }
            }
          }
          frame "角度标定" {
            n159 = global read "Global.vi" "产品型号"() -> (w181:string)
            n160 = case shown="\"R567B\"" w181 {
              tunnel: ["扭矩标定" w184 w208] -> w182
              frame Default {
              }
              frame "R567X" {
                n161 = disable-structure shown="启用" {
                  disable-tunnel: [w185 "扭矩标定" ("STEP")] -> w184
                  frame Disabled {
                    n162 = while {
                      tunnel: [w186] -> w185
                      stop <- w188 stop-if-true
                      n163 = Wait Until Next ms Multiple(millisecond multiple=u32 100 ("毫秒倍数")) -> ()  [unwired: 1 out]
                      n164 = call "R567X_CAN高级功能.vi"("Function"=T5."角度标定") -> ("完成"=w190:bool)  [unwired: 8 in, 6 out]
                      n165 = case shown="假" w190 {
                        tunnel: [w204 T4."Center Button" ("Which Button?")] -> w189
                        frame False {
                          n166 = global read "Global.vi" "Log"() -> (w198:string)
                          n167 = Concatenate Strings("角度标定失败！\nLOG>>>>>>>" ("message"), "\n", w198) -> (w197:string)
                          n168 = call <vilib>:"Three Button Dialog.vi"("Allow user to close window? (TRUE)"=FALSE, "Right Button Text (\"Cancel\")"="退出" ("Right Button Text (\"Cancel\")"), "Center Button Text (\"No\")"="忽略" ("Center Button Text (\"No\")"), "Left Button Text (\"Yes\")"="重试" ("Left Button Text (\"Yes\")"), "message"=w197) -> ("Which Button?"=w204:T4)  [unwired: 6 in]
                        }
                        frame True {
                        }
                      }
                      n169 = case shown="\"Center Button\"" w189 {
                        tunnel: [FALSE TRUE TRUE] -> w188
                        tunnel: [_ "扭矩标定" ("STEP") "退出自动" ("STEP")] -> w186
                        frame "Left Button", Default {
                        }
                        frame "Center Button" {
                        }
                        frame "Right Button" {
                        }
                      }
                    }
                  }
                  frame Enabled {
                  }
                }
              }
              frame "R567B" {
                n170 = disable-structure shown="启用" {
                  disable-tunnel: [w209 "扭矩标定" ("STEP")] -> w208
                  frame Disabled {
                    n171 = while {
                      tunnel: [w212] -> w209
                      stop <- w214 stop-if-true
                      n172 = Wait Until Next ms Multiple(millisecond multiple=u32 100 ("毫秒倍数")) -> ()  [unwired: 1 out]
                      n173 = call "R567B_CAN高级功能.vi"("Function"=T6."角度标定") -> ("完成"=w211:bool)  [unwired: 8 in, 6 out]
                      n174 = case shown="真" w211 {
                        tunnel: [w228 T4."Center Button" ("Which Button?")] -> w215
                        frame False {
                          n175 = global read "Global.vi" "Log"() -> (w222:string)
                          n176 = Concatenate Strings("角度标定失败！\nLOG>>>>>>>" ("message"), "\n", w222) -> (w221:string)
                          n177 = call <vilib>:"Three Button Dialog.vi"("Allow user to close window? (TRUE)"=FALSE, "Right Button Text (\"Cancel\")"="退出" ("Right Button Text (\"Cancel\")"), "Center Button Text (\"No\")"="忽略" ("Center Button Text (\"No\")"), "Left Button Text (\"Yes\")"="重试" ("Left Button Text (\"Yes\")"), "message"=w221) -> ("Which Button?"=w228:T4)  [unwired: 6 in]
                        }
                        frame True {
                        }
                      }
                      n178 = case shown="\"Center Button\"" w215 {
                        tunnel: [FALSE TRUE TRUE] -> w214
                        tunnel: [_ "扭矩标定" ("STEP") "退出自动" ("STEP")] -> w212
                        frame "Left Button", Default {
                        }
                        frame "Center Button" {
                        }
                        frame "Right Button" {
                        }
                      }
                    }
                  }
                  frame Enabled {
                  }
                }
              }
            }
            n179 = local write "STEP"(w182) -> ()
          }
          frame "角度标定2" {
            n180 = global read "Global.vi" "产品型号"() -> (w232:string)
            n181 = case shown="\"R567X\"" w232 {
              tunnel: ["套输入轴花键" w235] -> w233
              frame Default {
              }
              frame "R567X" {
                n182 = disable-structure shown="启用" {
                  disable-tunnel: [w236 "套输入轴花键"] -> w235
                  frame Disabled {
                    n183 = while {
                      tunnel: [w237] -> w236
                      stop <- w239 stop-if-true
                      n184 = Wait Until Next ms Multiple(millisecond multiple=u32 100 ("毫秒倍数")) -> ()  [unwired: 1 out]
                      n185 = call "R567X_CAN高级功能.vi"("Function"=T5."角度标定") -> ("完成"=w241:bool)  [unwired: 8 in, 6 out]
                      n186 = case shown="假" w241 {
                        tunnel: [w255 T4."Center Button" ("Which Button?")] -> w240
                        frame False {
                          n187 = global read "Global.vi" "Log"() -> (w249:string)
                          n188 = Concatenate Strings("角度标定失败！\nLOG>>>>>>>" ("message"), "\n", w249) -> (w248:string)
                          n189 = call <vilib>:"Three Button Dialog.vi"("Allow user to close window? (TRUE)"=FALSE, "Right Button Text (\"Cancel\")"="退出" ("Right Button Text (\"Cancel\")"), "Center Button Text (\"No\")"="忽略" ("Center Button Text (\"No\")"), "Left Button Text (\"Yes\")"="重试" ("Left Button Text (\"Yes\")"), "message"=w248) -> ("Which Button?"=w255:T4)  [unwired: 6 in]
                        }
                        frame True {
                        }
                      }
                      n190 = case shown="\"Right Button\"" w240 {
                        tunnel: [FALSE TRUE TRUE] -> w239
                        tunnel: [_ "套输入轴花键" ("STEP") "退出自动" ("STEP")] -> w237
                        frame "Left Button", Default {
                        }
                        frame "Center Button" {
                        }
                        frame "Right Button" {
                        }
                      }
                    }
                  }
                  frame Enabled {
                  }
                }
              }
            }
            n191 = local write "STEP"(w233) -> ()
          }
          frame "扭矩标定" {
            n192 = global read "Global.vi" "产品型号"() -> (w259:string)
            n193 = case shown="\"R567X\"" w259 {
              tunnel: ["试验项" ("STEP") w262] -> w260
              frame Default {
              }
              frame "R567X" {
                n194 = while {
                  tunnel: [w263] -> w262
                  stop <- w265 stop-if-true
                  n195 = Wait Until Next ms Multiple(millisecond multiple=u32 100 ("毫秒倍数")) -> ()  [unwired: 1 out]
                  n196 = call "R567X_CAN高级功能.vi"("Function"=T5."扭矩标定") -> ("完成"=w267:bool)  [unwired: 8 in, 6 out]
                  n197 = case shown="假" w267 {
                    tunnel: [w281 T4."Center Button" ("Which Button?")] -> w266
                    frame False {
                      n198 = global read "Global.vi" "Log"() -> (w277:string)
                      n199 = Concatenate Strings("扭矩标定失败！\nLOG>>>>>>>" ("message"), "\n", w277) -> (w274:string)
                      n200 = call <vilib>:"Three Button Dialog.vi"("Allow user to close window? (TRUE)"=FALSE, "Right Button Text (\"Cancel\")"="退出" ("Right Button Text (\"Cancel\")"), "Center Button Text (\"No\")"="忽略" ("Center Button Text (\"No\")"), "Left Button Text (\"Yes\")"="重试" ("Left Button Text (\"Yes\")"), "message"=w274) -> ("Which Button?"=w281:T4)  [unwired: 6 in]
                    }
                    frame True {
                    }
                  }
                  n201 = case shown="\"Center Button\"" w266 {
                    tunnel: [FALSE TRUE TRUE] -> w265
                    tunnel: [_ "试验项" ("STEP") "退出自动" ("STEP")] -> w263
                    frame "Left Button", Default {
                    }
                    frame "Center Button" {
                    }
                    frame "Right Button" {
                    }
                  }
                }
              }
            }
            n202 = local write "STEP"(w260) -> ()
          }
          frame "试验项" {
            n203 = global read "A180648.vi" "当前检测项"() -> (w284:T3)
            n204 = case shown="\"空载\", 默认" w284 {
              selector: w284 -> [w286 _]
              tunnel: [w289 "退输入轴花键" ("STEP")] -> w285
              frame "空载", Default {
                n205 = global read "Global.vi" "试验项目"() -> (w287:bool[])
                n206 = Index Array(array=w287, index=w286) -> (element=w288:bool)
                n207 = case shown="真" w288 {
                  tunnel: ["试验项" ("字符串") w296] -> w289
                  tunnel: w286 -> [_ w297]
                  frame False {
                    n208 = global read "A180648.vi" "当前检测项"() -> (w294:T3)
                    n209 = Increment(x=w294) -> (x+1=w293:T3)
                    n210 = global write "A180648.vi" "当前检测项"(w293) -> ()
                    n211 = local read "判定结果"() -> (w290:bool[][])
                    n212 = Build Array (concatenate)(w290, bool[] [FALSE] ("判定结果")) -> (w291:bool[][])
                    n213 = local write "判定结果"(w291) -> ()
                  }
                  frame True {
                    n214 = case shown="\"力特性\"" w297 {
                      tunnel: ["套输入轴花键" ("STEP") "套输入轴花键" ("STEP") "套输入轴花键" ("STEP") "套输入轴花键" ("STEP") w340 w343 "退输入轴花键" ("STEP") "退输入轴花键" ("STEP")] -> w296
                      frame "空载", Default {
                        n215 = call "浮动通知.vi"("通知内容"="空载试验") -> ()  [unwired: 11 in]
                        n216 = property on="试验项目" class="TabCtl (严格)"("Val(Sgnl)"=T1."空载" ("值(信号)")) -> ()  [unwired: 2 in, 2 out]
                      }
                      frame "功能" {
                        n217 = call "浮动通知.vi"("通知内容"="功能试验") -> ()  [unwired: 11 in]
                        n218 = property on="试验项目" class="TabCtl (严格)"("Val(Sgnl)"=T1."功能" ("值(信号)")) -> ()  [unwired: 2 in, 2 out]
                        n219 = global write "A180648.vi" "当前车速"(u16 20 ("当前车速")) -> ()
                      }
                      frame "力特性" {
                        n220 = global read "A180648.vi" "力特性参数"() -> (w306:sgl[])
                        n221 = call "浮动通知.vi"("通知内容"="力特性试验") -> ()  [unwired: 11 in]
                        n222 = for {
                          tunnel: w306 -> [w309] mode=indexing
                          i -> [w312]
                          w317 = u16 2 items=["byte", "word", "Dword"] ("数据类型")
                          w319 = u8 132 items=["I/O (P)"=128, "Input (I)"=129, "Output (Q)"=130, "Bit Memory (M)"=131, "Data (DB)"=132, "Instance Data (DI)"=133, "Local Data (L)"=134, "Predecessor Local Data (VL)"=135] ("寄存器类型")
                          n223 = Type Cast(type=u32 0 ("写入地址"), x=w309) -> (*(type *) &x=w315:u32)
                          n224 = Multiply(x=w312, y=4) -> (x*y=w313:i32)
                          n225 = Add(x=u32 152 ("写入地址"), y=w313) -> (x+y=w310:u32)
                          n226 = call "Write_Data.vi"("DB #"=u16 7, "寄存器类型"=w319, "写入数据"=w315, "数据类型"=w317, "写入地址"=w310) -> ()  [unwired: 4 in, 3 out]
                        }
                        n227 = property on="试验项目" class="TabCtl (严格)"("Val(Sgnl)"=T1."力特性" ("值(信号)")) -> ()  [unwired: 2 in, 2 out]
                      }
                      frame "传感器特性" {
                        n228 = property on="试验项目" class="TabCtl (严格)"("Val(Sgnl)"=T1."传感器特性" ("值(信号)")) -> ()  [unwired: 2 in, 2 out]
                        n229 = for {
                          tunnel: sgl[] [1.0, 15.0] ("力特性参数") -> [w324] mode=indexing
                          i -> [w327]
                          w332 = u16 2 items=["byte", "word", "Dword"] ("数据类型")
                          w334 = u8 132 items=["I/O (P)"=128, "Input (I)"=129, "Output (Q)"=130, "Bit Memory (M)"=131, "Data (DB)"=132, "Instance Data (DI)"=133, "Local Data (L)"=134, "Predecessor Local Data (VL)"=135] ("寄存器类型")
                          n230 = Type Cast(type=u32 0 ("写入地址"), x=w324) -> (*(type *) &x=w330:u32)
                          n231 = Multiply(x=w327, y=4) -> (x*y=w328:i32)
                          n232 = Add(x=u32 152 ("写入地址"), y=w328) -> (x+y=w325:u32)
                          n233 = call "Write_Data.vi"("DB #"=u16 7, "寄存器类型"=w334, "写入数据"=w330, "数据类型"=w332, "写入地址"=w325) -> ()  [unwired: 4 in, 3 out]
                        }
                        n234 = call "浮动通知.vi"("通知内容"="传感器特性试验") -> ()  [unwired: 11 in]
                      }
                      frame "电流特性" {
                        n235 = global read "Global.vi" "试验项目"() -> (w337:bool[])
                        n236 = call "浮动通知.vi"("通知内容"="电流特性试验") -> ()  [unwired: 11 in]
                        n237 = property on="试验项目" class="TabCtl (严格)"("Val(Sgnl)"=T1."电流特性" ("值(信号)")) -> ()  [unwired: 2 in, 2 out]
                        n238 = Index Array(array=w337, index=2 ("索引")) -> (element=w335:bool)
                        n239 = case shown="假" w335 {
                          tunnel: ["套输入轴花键" ("STEP") "判定" ("STEP")] -> w340
                          frame False {
                          }
                          frame True {
                          }
                        }
                      }
                      frame "振动NVH" {
                        n240 = call "浮动通知.vi"("通知内容"="振动NVH试验") -> ()  [unwired: 11 in]
                        n241 = property on="试验项目" class="TabCtl (严格)"("Val(Sgnl)"=T1."振动NVH" ("值(信号)")) -> ()  [unwired: 2 in, 2 out]
                        n242 = local read "NVH"() -> (w346:bool)
                        n243 = Select(t="判定" ("STEP"), s=w346, f="退输入轴花键" ("STEP")) -> (s? t:f=w343:string)
                      }
                      frame "逆向空载" {
                        n244 = global read "A180648.vi" "逆向空载参数"() -> (w351:string[][])
                        n245 = Index Array(array=w351, index (col)=1 ("禁用的索引 (列)")) -> (element=w350:string[])  [unwired: 1 in]
                        n246 = call "浮动通知.vi"("通知内容"="逆向空载试验") -> ()  [unwired: 11 in]
                        n247 = property on="试验项目" class="TabCtl (严格)"("Val(Sgnl)"=T1."逆向空载" ("值(信号)")) -> ()  [unwired: 2 in, 2 out]
                        n248 = for {
                          tunnel: w350 -> [w363] mode=indexing
                          i -> [w357]
                          w365 = u16 2 items=["byte", "word", "Dword"] ("数据类型")
                          w367 = u8 132 items=["I/O (P)"=128, "Input (I)"=129, "Output (Q)"=130, "Bit Memory (M)"=131, "Data (DB)"=132, "Instance Data (DI)"=133, "Local Data (L)"=134, "Predecessor Local Data (VL)"=135] ("寄存器类型")
                          n249 = Fract/Exp String To Number(string=w363, default (0 dbl)=sgl 0.0) -> (number=w361:sgl)  [unwired: 2 in, 1 out]
                          n250 = Multiply(x=w357, y=4) -> (x*y=w358:i32)
                          n251 = Add(x=u32 168 ("写入地址"), y=w358) -> (x+y=w355:u32)
                          n252 = Type Cast(type=u32 0 ("写入地址"), x=w361) -> (*(type *) &x=w360:u32)
                          n253 = call "Write_Data.vi"("DB #"=u16 7, "寄存器类型"=w367, "写入数据"=w360, "数据类型"=w365, "写入地址"=w355) -> ()  [unwired: 4 in, 3 out]
                        }
                      }
                      frame "磨合" {
                        n254 = global read "A180648.vi" "磨合参数"() -> (w370:string[][])
                        n255 = call "浮动通知.vi"("通知内容"="磨合") -> ()  [unwired: 11 in]
                        n256 = property on="试验项目" class="TabCtl (严格)"("Val(Sgnl)"=T1."磨合" ("值(信号)")) -> ()  [unwired: 2 in, 2 out]
                        n257 = Index Array(array=w370, index (col)=1 ("禁用的索引 (列)")) -> (element=w369:string[])  [unwired: 1 in]
                        n258 = for {
                          tunnel: w369 -> [w382] mode=indexing
                          i -> [w376]
                          w384 = u16 2 items=["byte", "word", "Dword"] ("数据类型")
                          w386 = u8 132 items=["I/O (P)"=128, "Input (I)"=129, "Output (Q)"=130, "Bit Memory (M)"=131, "Data (DB)"=132, "Instance Data (DI)"=133, "Local Data (L)"=134, "Predecessor Local Data (VL)"=135] ("寄存器类型")
                          n259 = Fract/Exp String To Number(string=w382, default (0 dbl)=sgl 0.0) -> (number=w380:sgl)  [unwired: 2 in, 1 out]
                          n260 = Multiply(x=w376, y=4) -> (x*y=w377:i32)
                          n261 = Add(x=u32 168 ("写入地址"), y=w377) -> (x+y=w374:u32)
                          n262 = Type Cast(type=u32 0 ("写入地址"), x=w380) -> (*(type *) &x=w379:u32)
                          n263 = call "Write_Data.vi"("DB #"=u16 7, "寄存器类型"=w386, "写入数据"=w379, "数据类型"=w384, "写入地址"=w374) -> ()  [unwired: 4 in, 3 out]
                        }
                      }
                    }
                  }
                }
              }
              frame "完成" {
              }
            }
            n264 = local write "STEP"(w285) -> ()
          }
          frame "判定" {
            n265 = stacked-sequence {
              frame #0 {
                n266 = global read "A180648.vi" "当前检测项"() -> (w388:T3)
                n267 = case shown="\"振动NVH\"" w388 {
                  frame "完成", Default {
                  }
                  frame "空载" {
                    n268 = global read "判定参数.vi" "空载判定参数"() -> (w400:T9)
                    n269 = global read "Global.vi" "Result"() -> (w399:refnum<vi>)
                    n270 = local read "空载试验"() -> (w401:cluster{dbl[], dbl[]}[])
                    n271 = call "空载试验判定.vi"("Result"=w399, "判定参数"=w400, "XY曲线"=w401) -> ("判定项长度"=w389:i32, "OK？"=w390:bool)  [unwired: 7 in]
                    n272 = global read "A180648.vi" "LED-空载"() -> (w395:refnum<vi>)
                    n273 = local read "判定结果"() -> (w391:bool[][])
                    n274 = Select(t=cluster{u32, u32}[] [{6618880, 6618880}, {6618880, 6618880}, {6618880, 6618880}, {6618880, 6618880}] ("颜色[4]"), s=w390, f=cluster{u32, u32}[] [{16711680, 16711680}, {16711680, 16711680}, {16711680, 16711680}, {16711680, 16711680}] ("颜色[4]")) -> (s? t:f=w396:cluster{u32, u32}[])
                    n275 = Build Array(TRUE, w390) -> (w394:bool[])
                    n276 = global write "判定参数.vi" "空载判定长度"(w389) -> ()
                    n277 = property class="Bool"(reference=w395, "Colors [4]"=w396) -> ()  [unwired: 1 in, 2 out]
                    n278 = Build Array (concatenate)(w391, w394) -> (w392:bool[][])
                    n279 = local write "判定结果"(w392) -> ()
                  }
                  frame "功能" {
                    n280 = global read "判定参数.vi" "功能判定参数"() -> (w414:T10)
                    n281 = local read "功能试验"() -> (w415:cluster{dbl[], dbl[]}[])
                    n282 = global read "Global.vi" "Result"() -> (w413:refnum<vi>)
                    n283 = call "功能试验判定.vi"("Result"=w413, "判定参数"=w414, "XY曲线"=w415) -> ("判定项长度"=w403:i32, "OK？"=w404:bool)  [unwired: 7 in]
                    n284 = global read "A180648.vi" "LED-功能"() -> (w409:refnum<vi>)
                    n285 = local read "判定结果"() -> (w405:bool[][])
                    n286 = Select(t=cluster{u32, u32}[] [{6618880, 6618880}, {6618880, 6618880}, {6618880, 6618880}, {6618880, 6618880}] ("颜色[4]"), s=w404, f=cluster{u32, u32}[] [{16711680, 16711680}, {16711680, 16711680}, {16711680, 16711680}, {16711680, 16711680}] ("颜色[4]")) -> (s? t:f=w410:cluster{u32, u32}[])
                    n287 = global write "判定参数.vi" "功能判定长度"(w403) -> ()
                    n288 = Build Array(TRUE, w404) -> (w408:bool[])
                    n289 = property class="Bool"(reference=w409, "Colors [4]"=w410) -> ()  [unwired: 1 in, 2 out]
                    n290 = Build Array (concatenate)(w405, w408) -> (w406:bool[][])
                    n291 = local write "判定结果"(w406) -> ()
                    "NVH" <- TRUE
                  }
                  frame "力特性" {
                    n292 = global read "判定参数.vi" "力特性判定参数"() -> (w418:T11)
                    n293 = local read "力特性试验"() -> (w428:cluster{dbl[], dbl[]}[])
                    n294 = for {
                      tunnel: w428 -> [w434]
                      tunnel: [w432] -> w419 mode=indexing
                      tunnel: w418 -> [w431] mode=indexing
                      tunnel: [w429] -> w416 mode=indexing
                      i -> [w430]
                      n295 = global read "Global.vi" "Result"() -> (w433:refnum<vi>)
                      n296 = call "力特性判定.vi"("Result"=w433, "索引"=w430, "判定参数"=w431, "XY曲线"=w434) -> ("判定项长度"=w429:i32, "OK？"=w432:bool)  [unwired: 6 in]
                    }
                    n297 = And Array Elements(Boolean array=w419) -> (logical AND=w417:bool)
                    n298 = global read "A180648.vi" "LED-力特性"() -> (w426:refnum<vi>)
                    n299 = local read "判定结果"() -> (w420:bool[][])
                    n300 = global write "判定参数.vi" "力特性判定长度"(w416) -> ()
                    n301 = Select(t=cluster{u32, u32}[] [{6618880, 6618880}, {6618880, 6618880}, {6618880, 6618880}, {6618880, 6618880}] ("颜色[4]"), s=w417, f=cluster{u32, u32}[] [{16711680, 16711680}, {16711680, 16711680}, {16711680, 16711680}, {16711680, 16711680}] ("颜色[4]")) -> (s? t:f=w427:cluster{u32, u32}[])
                    n302 = Build Array(TRUE, w417) -> (w423:bool[])
                    n303 = property class="Bool"(reference=w426, "Colors [4]"=w427) -> ()  [unwired: 1 in, 2 out]
                    n304 = Build Array (concatenate)(w420, w423) -> (w421:bool[][])
                    n305 = local write "判定结果"(w421) -> ()
                  }
                  frame "传感器特性" {
                    n306 = global read "判定参数.vi" "传感器特性判定参数"() -> (w446:T12)
                    n307 = local read "传感器特性试验"() -> (w447:cluster{dbl[], dbl[]}[])
                    n308 = global read "Global.vi" "Result"() -> (w445:refnum<vi>)
                    n309 = global read "A180648.vi" "LED-传感器特性"() -> (w441:refnum<vi>)
                    n310 = call "传感器特性判定.vi"("Result"=w445, "判定参数"=w446, "XY曲线"=w447) -> ("判定项长度"=w435:i32, "OK？"=w436:bool)  [unwired: 7 in]
                    n311 = local read "判定结果"() -> (w437:bool[][])
                    n312 = Select(t=cluster{u32, u32}[] [{6618880, 6618880}, {6618880, 6618880}, {6618880, 6618880}, {6618880, 6618880}] ("颜色[4]"), s=w436, f=cluster{u32, u32}[] [{16711680, 16711680}, {16711680, 16711680}, {16711680, 16711680}, {16711680, 16711680}] ("颜色[4]")) -> (s? t:f=w442:cluster{u32, u32}[])
                    n313 = Build Array(TRUE, w436) -> (w440:bool[])
                    n314 = global write "判定参数.vi" "传感器特性判定长度"(w435) -> ()
                    n315 = property class="Bool"(reference=w441, "Colors [4]"=w442) -> ()  [unwired: 1 in, 2 out]
                    n316 = Build Array (concatenate)(w437, w440) -> (w438:bool[][])
                    n317 = local write "判定结果"(w438) -> ()
                  }
                  frame "电流特性" {
                    n318 = global read "判定参数.vi" "电流特性判定参数"() -> (w453:T13)
                    n319 = local read "电流特性试验"() -> (w460:cluster{dbl[], dbl[]}[])
                    n320 = for {
                      tunnel: w460 -> [w466]
                      tunnel: [w464] -> w454 mode=indexing
                      tunnel: w453 -> [w463] mode=indexing
                      tunnel: [w461] -> w448 mode=indexing
                      i -> [w462]
                      n321 = global read "Global.vi" "Result"() -> (w465:refnum<vi>)
                      n322 = call "电流特性判定.vi"("Result"=w465, "索引"=w462, "判定参数"=w463, "XY曲线"=w466) -> ("判定项长度"=w461:i32, "OK？"=w464:bool)  [unwired: 6 in]
                    }
                    n323 = And Array Elements(Boolean array=w454) -> (logical AND=w452:bool)
                    n324 = global read "A180648.vi" "LED-电流特性"() -> (w458:refnum<vi>)
                    n325 = local read "判定结果"() -> (w455:bool[][])
                    n326 = Select(t=cluster{u32, u32}[] [{6618880, 6618880}, {6618880, 6618880}, {6618880, 6618880}, {6618880, 6618880}] ("颜色[4]"), s=w452, f=cluster{u32, u32}[] [{16711680, 16711680}, {16711680, 16711680}, {16711680, 16711680}, {16711680, 16711680}] ("颜色[4]")) -> (s? t:f=w459:cluster{u32, u32}[])
                    n327 = global write "判定参数.vi" "电流特性判定长度"(w448) -> ()
                    n328 = Build Array(TRUE, w452) -> (w457:bool[])
                    n329 = property class="Bool"(reference=w458, "Colors [4]"=w459) -> ()  [unwired: 1 in, 2 out]
                    n330 = Build Array (concatenate)(w455, w457) -> (w456:bool[][])
                    n331 = local write "判定结果"(w456) -> ()
                  }
                  frame "振动NVH" {
                    n332 = local read "振动1NVH-FFT"() -> (w477:cluster{"f0":dbl, "df":dbl, "magnitude":dbl[]}[])
                    n333 = local read "振动2NHV-FFT"() -> (w476:cluster{"f0":dbl, "df":dbl, "magnitude":dbl[]}[])
                    n334 = global read "判定参数.vi" "振动判定范围"() -> (w473:T14)
                    n335 = global read "判定参数.vi" "振动判定"() -> (w474:T15)
                    n336 = global read "Global.vi" "Result"() -> (w483:refnum<vi>)
                    n337 = Build Array (concatenate)(w477, w476) -> (w475:cluster{"f0":dbl, "df":dbl, "magnitude":dbl[]}[])
                    n338 = global read "A180648.vi" "LED-振动NVH"() -> (w484:refnum<vi>)
                    n339 = call "振动判定.vi"("Result"=w483, "振动判定"=w474, "振动判定范围"=w473, "FFT"=w475) -> ("判定项长度"=w470:i32, "Limit Specifications"=w472:cluster{"x0":dbl, "dx":dbl, "Y":dbl[]}[][], "FFT 2"=w471:cluster{"f0":dbl, "df":dbl, "magnitude":dbl[]}[], "OK？"=w478:bool)  [unwired: 4 in]
                    n340 = Select(t=cluster{u32, u32}[] [{6618880, 6618880}, {6618880, 6618880}, {6618880, 6618880}, {6618880, 6618880}] ("颜色[4]"), s=w478, f=cluster{u32, u32}[] [{16711680, 16711680}, {16711680, 16711680}, {16711680, 16711680}, {16711680, 16711680}] ("颜色[4]")) -> (s? t:f=w486:cluster{u32, u32}[])
                    n341 = for {
                      tunnel: w472 -> [w490] mode=indexing
                      tunnel: w471 -> [w489] mode=indexing
                      tunnel: [w488] -> w469 mode=indexing
                      n342 = Build Array (concatenate)(w489, w490) -> (w488:cluster{"x0":dbl, "dx":dbl, "Y":dbl[]}[])
                    }
                    n343 = global write "判定参数.vi" "振动判定长度"(w470) -> ()
                    n344 = property class="Bool"(reference=w484, "Colors [4]"=w486) -> ()  [unwired: 1 in, 2 out]
                    n345 = local read "判定结果"() -> (w479:bool[][])
                    n346 = Build Array(TRUE, w478) -> (w482:bool[])
                    n347 = Index Array(array=w469) -> (element #1=w468:cluster{"x0":dbl, "dx":dbl, "Y":dbl[]}[], element #2=w467:cluster{"x0":dbl, "dx":dbl, "Y":dbl[]}[])  [unwired: 4 in]
                    n348 = Build Array (concatenate)(w479, w482) -> (w480:bool[][])
                    n349 = local write "振动1NVH-FFT"(w468) -> ()
                    n350 = local write "振动2NHV-FFT"(w467) -> ()
                    n351 = local write "判定结果"(w480) -> ()
                  }
                  frame "磨合" {
                    w491 = TRUE
                    n352 = global read "A180648.vi" "LED-磨合"() -> (w495:refnum<vi>)
                    n353 = property class="Bool"(reference=w495, "Colors [4]"=cluster{u32, u32}[] [{6618880, 6618880}, {6618880, 6618880}, {6618880, 6618880}, {6618880, 6618880}] ("颜色[4]")) -> ()  [unwired: 1 in, 2 out]
                    n354 = local read "判定结果"() -> (w492:bool[][])
                    n355 = Build Array(w491, w491) -> (w494:bool[])
                    n356 = Build Array (concatenate)(w492, w494) -> (w493:bool[][])
                    n357 = local write "判定结果"(w493) -> ()
                  }
                  frame "逆向空载" {
                    n358 = global read "判定参数.vi" "逆向空载判定参数"() -> (w508:T16)
                    n359 = local read "逆向空载试验"() -> (w509:cluster{dbl[], dbl[]}[])
                    n360 = global read "Global.vi" "Result"() -> (w507:refnum<vi>)
                    n361 = global read "A180648.vi" "LED-逆向空载"() -> (w503:refnum<vi>)
                    n362 = call "逆向空载试验判定.vi"("Result"=w507, "判定参数"=w508, "XY曲线"=w509) -> ("判定项长度"=w497:i32, "OK？"=w498:bool)  [unwired: 7 in]
                    n363 = Select(t=cluster{u32, u32}[] [{6618880, 6618880}, {6618880, 6618880}, {6618880, 6618880}, {6618880, 6618880}] ("颜色[4]"), s=w498, f=cluster{u32, u32}[] [{16711680, 16711680}, {16711680, 16711680}, {16711680, 16711680}, {16711680, 16711680}] ("颜色[4]")) -> (s? t:f=w504:cluster{u32, u32}[])
                    n364 = property class="Bool"(reference=w503, "Colors [4]"=w504) -> ()  [unwired: 1 in, 2 out]
                    n365 = global write "判定参数.vi" "逆向空载判定长度"(w497) -> ()
                    n366 = local read "判定结果"() -> (w500:bool[][])
                    n367 = Build Array(TRUE, w498) -> (w502:bool[])
                    n368 = Build Array (concatenate)(w500, w502) -> (w501:bool[][])
                    n369 = local write "判定结果"(w501) -> ()
                  }
                }
              }
              frame #1 {
                n370 = global read "A180648.vi" "当前检测项"() -> (w511:T3)
                n371 = Increment(x=w511) -> (x+1=w512:T3)
                n372 = local write "STEP"("试验项" ("STEP")) -> ()
                n373 = global write "A180648.vi" "当前检测项"(w512) -> ()
              }
            }
          }
          frame "套输入轴花键" {
            n374 = call "设备状态.vi"() -> ("Status_Read"=w513:i16)  [unwired: 11 in]
            n375 = case shown="103" w513 {
              frame 0, Default {
                n376 = call "设备状态.vi"("枚举"=enum16{"Read", "Write"}."Write", "Status_Write"=i16 102 ("设备状态")) -> ()  [unwired: 9 in, 1 out]
              }
              frame 103 {
                n377 = global read "A180648.vi" "当前检测项"() -> (w517:T3)
                n378 = case shown="\"力特性\"" w517 {
                  tunnel: ["退输出轴花键" ("STEP") "套输出轴花键" ("STEP") "套输出轴花键" ("STEP") "套输出轴花键" ("STEP") "套输出轴花键" ("STEP")] -> w516
                  frame "空载", Default {
                  }
                  frame "功能" {
                  }
                  frame "力特性" {
                  }
                  frame "传感器特性" {
                  }
                  frame "电流特性" {
                  }
                }
                n379 = local write "STEP"(w516) -> ()
              }
              frame 1024 {
                n380 = local write "STEP"("退出自动" ("STEP")) -> ()
              }
            }
          }
          frame "退输入轴花键" {
            n381 = call "设备状态.vi"() -> ("Status_Read"=w524:i16)  [unwired: 11 in]
            n382 = case shown="105" w524 {
              frame 0, Default {
                n383 = call "设备状态.vi"("枚举"=enum16{"Read", "Write"}."Write", "Status_Write"=i16 104 ("设备状态")) -> ()  [unwired: 9 in, 1 out]
              }
              frame 105 {
                n384 = global read "A180648.vi" "当前检测项"() -> (w528:T3)
                n385 = case shown="\"磨合\"" w528 {
                  tunnel: ["自动" ("STEP") "退输出轴花键" ("STEP") "套输出轴花键" ("STEP") "套输出轴花键" ("STEP") "退输出轴花键" ("STEP")] -> w527
                  frame Default {
                  }
                  frame "振动NVH" {
                  }
                  frame "逆向空载" {
                  }
                  frame "磨合" {
                  }
                  frame "完成" {
                  }
                }
                n386 = local write "STEP"(w527) -> ()
              }
              frame 1024 {
                n387 = local write "STEP"("退出自动" ("STEP")) -> ()
              }
            }
          }
          frame "套输出轴花键" {
            n388 = call "设备状态.vi"() -> ("Status_Read"=w535:i16)  [unwired: 11 in]
            n389 = case shown="107" w535 {
              frame 0, Default {
                n390 = call "设备状态.vi"("枚举"=enum16{"Read", "Write"}."Write", "Status_Write"=i16 106 ("设备状态")) -> ()  [unwired: 9 in, 1 out]
              }
              frame 107 {
                n391 = local write "STEP"("设置输出轴模式" ("STEP")) -> ()
              }
              frame 1024 {
                n392 = local write "STEP"("退出自动" ("STEP")) -> ()
              }
            }
          }
          frame "退输出轴花键" {
            n393 = call "设备状态.vi"() -> ("Status_Read"=w540:i16)  [unwired: 11 in]
            n394 = case shown="109" w540 {
              frame 0, Default {
                n395 = call "设备状态.vi"("枚举"=enum16{"Read", "Write"}."Write", "Status_Write"=i16 108 ("设备状态")) -> ()  [unwired: 9 in, 1 out]
              }
              frame 109 {
                n396 = global read "A180648.vi" "当前检测项"() -> (w543:T3)
                n397 = case shown="\"空载\"" w543 {
                  tunnel: ["自动" ("STEP") "自动" ("STEP") "报表" ("STEP") "自动" ("STEP")] -> w544
                  frame Default {
                  }
                  frame "振动NVH" {
                    n398 = call "设备状态.vi"("枚举"=enum16{"Read", "Write"}."Write", "Status_Write"=i16 142 ("设备状态")) -> ()  [unwired: 9 in, 1 out]
                  }
                  frame "完成" {
                    n399 = call "浮动通知.vi"("通知内容"="检测完成！" ("Status")) -> ()  [unwired: 11 in]
                    n400 = call "设备状态.vi"("枚举"=enum16{"Read", "Write"}."Write", "Status_Write"=i16 160) -> ()  [unwired: 9 in, 1 out]
                  }
                  frame "空载" {
                    n401 = call "设备状态.vi"("枚举"=enum16{"Read", "Write"}."Write", "Status_Write"=i16 112) -> ()  [unwired: 9 in, 1 out]
                  }
                }
                n402 = local write "STEP"(w544) -> ()
              }
              frame 110 {
                n403 = local write "STEP"("退出自动" ("STEP")) -> ()
              }
            }
          }
          frame "设置输出轴模式" {
            n404 = global read "A180648.vi" "当前检测项"() -> (w558:T3)
            n405 = case shown="\"力特性\"" w558 {
              tunnel: ["自动" ("STEP") "自动" ("STEP") "自动" ("STEP") "自动" ("STEP") "自动" ("STEP") "自动" ("STEP") "自动" ("STEP")] -> w557
              frame Default {
                n406 = call-poly "模式选择.vi"("Max Torque"=200.0, "Velocity"=sgl 0.0) -> ()  [unwired: 9 in, 1 out]
              }
              frame "功能" {
                n407 = stacked-sequence {
                  frame #0 {
                    n408 = call "设备状态.vi"("枚举"=enum16{"Read", "Write"}."Write", "Status_Write"=i16 122 ("设备状态")) -> ()  [unwired: 9 in, 1 out]
                  }
                  frame #1 {
                    n409 = Wait (ms)(milliseconds to wait=u32 500 ("等待时间（毫秒）")) -> ()  [unwired: 1 out]
                  }
                  frame #2 {
                    n410 = global read "A180648.vi" "功能试验参数"() -> (w569:T17)
                    n411 = Unbundle By Name(w569) -> ("负载扭矩"=w567:dbl)
                    n412 = Subtract(x=w567, y=19.0) -> (x-y=w566:dbl)
                    n413 = call-poly "模式选择.vi"("Max Torque"=w566) -> ()  [unwired: 10 in, 1 out]
                  }
                }
              }
              frame "力特性" {
                n414 = call "设备状态.vi"("枚举"=enum16{"Read", "Write"}."Write", "Status_Write"=i16 130 ("设备状态")) -> ()  [unwired: 9 in, 1 out]
                n415 = call-poly "模式选择.vi"() -> ()  [unwired: 11 in, 1 out]
              }
              frame "传感器特性" {
                n416 = call "设备状态.vi"("枚举"=enum16{"Read", "Write"}."Write", "Status_Write"=i16 130 ("设备状态")) -> ()  [unwired: 9 in, 1 out]
                n417 = call-poly "模式选择.vi"() -> ()  [unwired: 11 in, 1 out]
              }
              frame "逆向空载" {
                n418 = call "设备状态.vi"("枚举"=enum16{"Read", "Write"}."Write", "Status_Write"=i16 152 ("设备状态")) -> ()  [unwired: 9 in, 1 out]
              }
              frame "磨合" {
                n419 = call "设备状态.vi"("枚举"=enum16{"Read", "Write"}."Write", "Status_Write"=i16 152 ("设备状态")) -> ()  [unwired: 9 in, 1 out]
              }
              frame "电流特性" {
                n420 = call "设备状态.vi"("枚举"=enum16{"Read", "Write"}."Write", "Status_Write"=i16 130 ("设备状态")) -> ()  [unwired: 9 in, 1 out]
                n421 = call-poly "模式选择.vi"() -> ()  [unwired: 11 in, 1 out]
              }
            }
            n422 = local write "STEP"(w557) -> ()
          }
          frame "自动" {
            n423 = global read "Global.vi" "设备状态"() -> (w585:i16)
            n424 = case shown="124" w585 {
              frame -128 {
                n425 = call-poly "模式选择.vi"() -> ("error out"=w586:errorcluster)  [unwired: 11 in]
                n426 = global write "Global.vi" "计时开始"(FALSE ("计时开始")) -> ()
                n427 = call "浮动通知.vi"("通知内容"="复位中……" ("Status")) -> ()  [unwired: 11 in]
                n428 = call "SetActualPosition.vi"("error in (no error)"=w586) -> ()  [unwired: 10 in, 1 out]
              }
              frame Default {
              }
              frame 0 {
                n429 = global write "Global.vi" "计时开始"(FALSE ("计时开始")) -> ()
                n430 = call "浮动通知.vi"("通知内容"="手动状态！" ("Status")) -> ()  [unwired: 11 in]
              }
              frame 1 {
                n431 = call "浮动通知.vi"("通知内容"="请复位！" ("Status")) -> ()  [unwired: 11 in]
              }
              frame 5 {
                n432 = call "浮动通知.vi"("通知内容"="复位完成" ("Status")) -> ()  [unwired: 11 in]
                n433 = global write "Global.vi" "计时开始"(FALSE ("计时开始")) -> ()
              }
              frame 8 {
                n434 = call "浮动通知.vi"("通知内容"="程序停止！" ("Status")) -> ()  [unwired: 11 in]
              }
              frame 100 {
                n435 = call "浮动通知.vi"("通知内容"="请放入产品后按启动夹紧产品！" ("Status")) -> ()  [unwired: 11 in]
              }
              frame 101 {
                n436 = local write "STEP"("扫码" ("STEP")) -> ()
              }
              frame 112 {
                n437 = global read "System_Conf.vi" "system"() -> (w600:T8)
                n438 = call "传感器数据.vi"() -> ("传感器读数"=w607:T18)  [unwired: 11 in]
                n439 = Unbundle By Name(w607) -> ("输入旋转位移"=w606:sgl, "输入扭矩"=w599:sgl)
                n440 = Unbundle By Name(w600) -> ("空载滤波"=w601:bool, "空载扭矩系数"=w604:dbl)
                n441 = local read "空载正向初始化"() -> (w602:bool)
                n442 = Multiply(x=w599, y=w604) -> (x*y=w603:dbl)
                n443 = case shown="真" w601 {
                  tunnel: w606 -> [w609 w615]
                  tunnel: w603 -> [w608 w614]
                  tunnel: [w609 w612] -> w597
                  tunnel: [w608 w611] -> w598
                  tunnel: w602 -> [_ w610]
                  frame False {
                  }
                  frame True {
                    w613 = 5 ("Averaging Size")
                    n444 = call-poly <userlib>:"MGI Running Average.vi"("Averaging Size"=w613, "Initialize? (F)"=w610, "Value"=w615) -> ("Average"=w612:sgl)  [unwired: 8 in]
                    n445 = call-poly <userlib>:"MGI Running Average.vi"("Averaging Size"=w613, "Initialize? (F)"=w610, "Value"=w614) -> ("Average"=w611:dbl)  [unwired: 8 in]
                  }
                }
                n446 = Greater Or Equal To 0?(x=w597) -> (x >= 0?=w605:bool)
                n447 = case shown="真" w605 {
                  tunnel: w597 -> [_ w617]
                  tunnel: w598 -> [_ w616]
                  frame False {
                  }
                  frame True {
                    n448 = control-ref of="空载试验"() -> (w621:refnum<vi>)
                    n449 = call "曲线采集.vi"("曲线引用"=w621, "曲线索引"=0, "X"=w617, "Y"=w616) -> ("错误输出"=w619:errorcluster)  [unwired: 10 in, 1 out]
                    n450 = Unbundle By Name(w619) -> ("status"=w618:bool)
                    n451 = local write "空载正向初始化"(w618) -> ()
                  }
                }
              }
              frame 113 {
                n452 = call "设备状态.vi"("枚举"=enum16{"Read", "Write"}."Write", "Status_Write"=i16 114 ("设备状态")) -> ()  [unwired: 9 in, 1 out]
                n453 = local write "STEP"("等待" ("STEP")) -> ()
              }
              frame 114 {
                n454 = global read "System_Conf.vi" "system"() -> (w629:T8)
                n455 = call "传感器数据.vi"() -> ("传感器读数"=w636:T18)  [unwired: 11 in]
                n456 = Unbundle By Name(w636) -> ("输入旋转位移"=w635:sgl, "输入扭矩"=w634:sgl)
                n457 = Unbundle By Name(w629) -> ("空载滤波"=w628:bool, "空载扭矩系数"=w626:dbl)
                n458 = local read "空载逆向初始化"() -> (w625:bool)
                n459 = Multiply(x=w634, y=w626) -> (x*y=w627:dbl)
                n460 = case shown="真" w628 {
                  tunnel: w635 -> [w640 w646]
                  tunnel: w627 -> [w639 w645]
                  tunnel: [w640 w643] -> w633
                  tunnel: [w639 w642] -> w632
                  tunnel: w625 -> [_ w641]
                  frame False {
                  }
                  frame True {
                    w644 = 10 ("Averaging Size")
                    n461 = call-poly <userlib>:"MGI Running Average.vi"("Averaging Size"=w644, "Initialize? (F)"=w641, "Value"=w646) -> ("Average"=w643:sgl)  [unwired: 8 in]
                    n462 = call-poly <userlib>:"MGI Running Average.vi"("Averaging Size"=w644, "Initialize? (F)"=w641, "Value"=w645) -> ("Average"=w642:dbl)  [unwired: 8 in]
                  }
                }
                n463 = control-ref of="空载试验"() -> (w638:refnum<vi>)
                n464 = call "曲线采集.vi"("曲线引用"=w638, "曲线索引"=1, "X"=w633, "Y"=w632) -> ("错误输出"=w631:errorcluster)  [unwired: 10 in, 1 out]
                n465 = Unbundle By Name(w631) -> ("status"=w630:bool)
                n466 = local write "空载逆向初始化"(w630) -> ()
              }
              frame 115 {
                n467 = local write "STEP"("判定" ("STEP")) -> ()
              }
              frame 122 {
                w651 = 1 ("Averaging Size")
                n468 = call "传感器数据.vi"() -> ("传感器读数"=w659:T18)  [unwired: 11 in]
                n469 = local read "功能正向初始化"() -> (w650:bool)
                n470 = Unbundle By Name(w659) -> ("输入旋转位移"=w657:sgl, "输入扭矩"=w655:sgl, "输出扭矩(大)"=w653:sgl)
                n471 = Add(x=w655, y=sgl 0.2) -> (x+y=w649:sgl)
                n472 = case shown="真" w650 {
                  frame False {
                  }
                  frame True {
                    n473 = vi-ref "NVH_TEST.vi"() -> (w664:refnum<vi>)
                    n474 = property class="VI"(reference=w664) -> (error out=w666:errorcluster, "Name"=w667:string)  [unwired: 1 in, 1 out]
                    n475 = control-ref of="振动2NHV-FFT"() -> (w660:refnum<vi>)
                    n476 = control-ref of="振动1NVH-FFT"() -> (w662:refnum<vi>)
                    n477 = Open VI Reference(type specifier VI Refnum (for type only)=refnum<vi> refnum, vi path=w667, options=128 ("调用并忽略输出"), error in (no error)=w666) -> (vi reference=w663:refnum<vi>)  [unwired: 2 in, 1 out]
                    n478 = call-by-ref "开始异步调用"(reference=w663, "振动NHV-FFT"=w660, "振动NVH-Order"=w662) -> (reference out=w670:refnum<vi>, error out=w668:errorcluster)  [unwired: 11 in]
                    n479 = Close Reference(reference=w670, error in (no error)=w668) -> (error out=w669:errorcluster)
                    n480 = call <vilib>:"Simple Error Handler.vi"("error in (no error)"=w669) -> ()  [unwired: 4 in, 5 out]
                  }
                }
                n481 = call-poly <userlib>:"MGI Running Average.vi"("Averaging Size"=w651, "Initialize? (F)"=w650, "Value"=w657) -> ("Average"=w656:sgl)  [unwired: 8 in]
                n482 = call-poly <userlib>:"MGI Running Average.vi"("Averaging Size"=w651, "Initialize? (F)"=w650, "Value"=w649) -> ("Average"=w654:sgl)  [unwired: 8 in]
                n483 = call-poly <userlib>:"MGI Running Average.vi"("Averaging Size"=w651, "Initialize? (F)"=w650, "Value"=w653) -> ("Average"=w652:sgl)  [unwired: 8 in]
                n484 = Greater Or Equal To 0?(x=w656) -> (x >= 0?=w658:bool)
                n485 = case shown="真" w658 {
                  tunnel: w654 -> [_ w677]
                  tunnel: w652 -> [_ w674]
                  tunnel: w656 -> [_ w673]
                  frame False {
                  }
                  frame True {
                    n486 = control-ref of="功能试验"() -> (w676:refnum<vi>)
                    n487 = call "曲线采集.vi"("曲线引用"=w676, "曲线索引"=0, "X"=w673, "Y"=w677) -> ("错误输出"=w672:errorcluster)  [unwired: 10 in, 1 out]
                    n488 = call "曲线采集.vi"("曲线引用"=w676, "曲线索引"=2, "X"=w673, "Y"=w674) -> ()  [unwired: 10 in, 2 out]
                    n489 = Unbundle By Name(w672) -> ("status"=w671:bool)
                    n490 = local write "功能正向初始化"(w671) -> ()
                  }
                }
              }
              frame 123 {
                n491 = stacked-sequence {
                  frame #0 {
                    n492 = call "设备状态.vi"("枚举"=enum16{"Read", "Write"}."Write", "Status_Write"=i16 124 ("设备状态")) -> ()  [unwired: 9 in, 1 out]
                  }
                  frame #1 {
                    n493 = global read "A180648.vi" "功能试验参数"() -> (w683:T17)
                    n494 = Unbundle By Name(w683) -> ("负载扭矩"=w682:dbl)
                    n495 = Subtract(x=19.0 ("y"), y=w682) -> (x-y=w684:dbl)
                    n496 = call-poly "模式选择.vi"("Max Torque"=w684) -> ()  [unwired: 10 in, 1 out]
                  }
                }
              }
              frame 124 {
                w692 = 1 ("Averaging Size")
                n497 = call "传感器数据.vi"() -> ("传感器读数"=w700:T18)  [unwired: 11 in]
                n498 = Unbundle By Name(w700) -> ("输入旋转位移"=w699:sgl, "输入扭矩"=w697:sgl, "输出扭矩(大)"=w695:sgl)
                n499 = control-ref of="功能试验"() -> (w690:refnum<vi>)
                n500 = local read "功能逆向初始化"() -> (w693:bool)
                n501 = Add(x=sgl 0.2, y=w697) -> (x+y=w686:sgl)
                n502 = call-poly <userlib>:"MGI Running Average.vi"("Averaging Size"=w692, "Initialize? (F)"=w693, "Value"=w686) -> ("Average"=w696:sgl)  [unwired: 8 in]
                n503 = call-poly <userlib>:"MGI Running Average.vi"("Averaging Size"=w692, "Initialize? (F)"=w693, "Value"=w695) -> ("Average"=w694:sgl)  [unwired: 8 in]
                n504 = call-poly <userlib>:"MGI Running Average.vi"("Averaging Size"=w692, "Initialize? (F)"=w693, "Value"=w699) -> ("Average"=w698:sgl)  [unwired: 8 in]
                n505 = call "曲线采集.vi"("曲线引用"=w690, "曲线索引"=1, "X"=w698, "Y"=w696) -> ("错误输出"=w688:errorcluster)  [unwired: 10 in, 1 out]
                n506 = call "曲线采集.vi"("曲线引用"=w690, "曲线索引"=3, "X"=w698, "Y"=w694) -> ()  [unwired: 10 in, 2 out]
                n507 = Unbundle By Name(w688) -> ("status"=w687:bool)
                n508 = local write "功能逆向初始化"(w687) -> ()
              }
              frame 125 {
                n509 = global write "Global.vi" "STOP_NVH"(TRUE ("STOP_NVH")) -> ()
                n510 = call-poly "模式选择.vi"() -> ()  [unwired: 11 in, 1 out]
                n511 = local write "STEP"("判定" ("STEP")) -> ()
              }
              frame 130 {
                w703 = TRUE
                n512 = global read "A180648.vi" "当前检测项"() -> (w705:T3)
                n513 = case shown="默认" w705 {
                  tunnel: [0 100] -> w704
                  frame Default {
                    w708 = u16 2 items=["byte", "word", "Dword"] ("数据类型")
                    w709 = u8 132 items=["I/O (P)"=128, "Input (I)"=129, "Output (Q)"=130, "Bit Memory (M)"=131, "Data (DB)"=132, "Instance Data (DI)"=133, "Local Data (L)"=134, "Predecessor Local Data (VL)"=135] ("寄存器类型")
                    n514 = global read "A180648.vi" "车速"() -> (w715:sgl[])
                    n515 = Index Array(array=w715) -> (element=w714:sgl)  [unwired: 1 in]
                    n516 = Round Toward +Infinity(x=w714) -> (ceil(x): smallest int >= x=w713:sgl)
                    n517 = disable-structure shown="禁用" {
                      frame Disabled {
                        n518 = call-poly "模式选择.vi"("Max Torque"=200.0, "Velocity"=sgl 1.0) -> ()  [unwired: 9 in, 1 out]
                      }
                      frame Enabled {
                      }
                    }
                    n519 = Type Cast(type=u32 0, x=w714) -> (*(type *) &x=w716:u32)
                    n520 = To Unsigned Word Integer(number=w713) -> (unsigned 16bit integer=w712:u16)
                    n521 = call "Write_Data.vi"("DB #"=u16 7, "寄存器类型"=w709, "写入数据"=w716, "数据类型"=w708, "写入地址"=u32 160) -> ()  [unwired: 4 in, 3 out]
                    n522 = global write "A180648.vi" "当前车速"(w712) -> ()
                  }
                  frame "传感器特性" {
                    w719 = u32 0
                    w721 = u16 2 items=["byte", "word", "Dword"] ("数据类型")
                    w724 = u8 132 items=["I/O (P)"=128, "Input (I)"=129, "Output (Q)"=130, "Bit Memory (M)"=131, "Data (DB)"=132, "Instance Data (DI)"=133, "Local Data (L)"=134, "Predecessor Local Data (VL)"=135] ("寄存器类型")
                    n523 = global write "A180648.vi" "当前车速"(w719) -> ()
                    n524 = call "Write_Data.vi"("DB #"=u16 7, "寄存器类型"=w724, "写入数据"=w719, "数据类型"=w721, "写入地址"=u32 160) -> ()  [unwired: 4 in, 3 out]
                    n525 = call-poly "模式选择.vi"() -> ()  [unwired: 11 in, 1 out]
                  }
                }
                n526 = local write "力特性逆向回程"(w703) -> ()
                n527 = local write "力特性正向去程"(w703) -> ()
                n528 = local write "力特性逆向去程"(w703) -> ()
                n529 = local write "力特性正向回程"(w703) -> ()
                n530 = local write "当前车速"(w704) -> ()
              }
              frame 132 {
                n531 = control-ref of="电流特性试验"() -> (w729:refnum<vi>)
                n532 = local read "当前车速"() -> (w726:i32)
                n533 = global read "Global.vi" "传感器读数"() -> (w725:T18)
                n534 = control-ref of="力特性试验"() -> (w727:refnum<vi>)
                n535 = control-ref of="传感器特性试验"() -> (w728:refnum<vi>)
                n536 = local read "力特性正向去程"() -> (w730:bool)
                n537 = case shown="0, 默认" w726 {
                  selector: w726 -> [w753 _]
                  tunnel: w725 -> [w758 w774]
                  tunnel: w727 -> [w757 _]
                  tunnel: w728 -> [_ w772]
                  tunnel: w729 -> [w755 _]
                  tunnel: w730 -> [w744 w760]
                  tunnel: [FALSE FALSE] -> w731
                  tunnel: [w745 w764] -> w732
                  tunnel: [w747 _] -> w733
                  tunnel: [w746 _] -> w734
                  tunnel: [_ w763] -> w735
                  tunnel: [_ w762] -> w736
                  tunnel: [_ w761] -> w737
                  tunnel: 10 -> [w743 w759]
                  frame 0, Default {
                    n538 = Unbundle By Name(w758) -> ("输入扭矩"=w756:sgl, "输出扭矩(大)"=w742:sgl, "吸收电流"=w754:sgl)
                    n539 = Multiply(x=w753, y=4) -> (x*y=w750:i32)
                    n540 = Subtract(x=w742, y=sgl -0.2) -> (x-y=w740:sgl)
                    n541 = call-poly <userlib>:"MGI Running Average.vi"("Averaging Size"=w743, "Initialize? (F)"=w744, "Value"=w754) -> ("Average"=w746:sgl)  [unwired: 8 in]
                    n542 = call-poly <userlib>:"MGI Running Average.vi"("Averaging Size"=w743, "Initialize? (F)"=w744, "Value"=w756) -> ("Average"=w745:sgl)  [unwired: 8 in]
                    n543 = call-poly <userlib>:"MGI Running Average.vi"("Averaging Size"=w743, "Initialize? (F)"=w744, "Value"=w740) -> ("Average"=w747:sgl)  [unwired: 8 in]
                    n544 = Add(x=w750, y=0) -> (x+y=w749:i32)
                    n545 = call "曲线采集.vi"("曲线引用"=w755, "曲线索引"=w749, "X"=w745, "Y"=w746) -> ()  [unwired: 10 in, 2 out]
                    n546 = call "曲线采集.vi"("曲线引用"=w757, "曲线索引"=w749, "X"=w745, "Y"=w747) -> ()  [unwired: 10 in, 2 out]
                  }
                  frame 100 {
                    n547 = Unbundle By Name(w774) -> ("输入扭矩"=w773:sgl)
                    n548 = call "占空比.vi"() -> ("T1+T2"=w769:dbl, "T2"=w770:dbl, "T1"=w771:dbl)  [unwired: 9 in]
                    n549 = call-poly <userlib>:"MGI Running Average.vi"("Averaging Size"=w759, "Initialize? (F)"=w760, "Value"=w773) -> ("Average"=w764:sgl)  [unwired: 8 in]
                    n550 = call-poly <userlib>:"MGI Running Average.vi"("Averaging Size"=w759, "Initialize? (F)"=w760, "Value"=w769) -> ("Average"=w763:dbl)  [unwired: 8 in]
                    n551 = call-poly <userlib>:"MGI Running Average.vi"("Averaging Size"=w759, "Initialize? (F)"=w760, "Value"=w771) -> ("Average"=w761:dbl)  [unwired: 8 in]
                    n552 = call-poly <userlib>:"MGI Running Average.vi"("Averaging Size"=w759, "Initialize? (F)"=w760, "Value"=w770) -> ("Average"=w762:dbl)  [unwired: 8 in]
                    n553 = call "曲线采集.vi"("曲线引用"=w772, "曲线索引"=2, "X"=w764, "Y"=w763) -> ()  [unwired: 10 in, 2 out]
                    n554 = call "曲线采集.vi"("曲线引用"=w772, "曲线索引"=0, "X"=w764, "Y"=w761) -> ()  [unwired: 10 in, 2 out]
                    n555 = call "曲线采集.vi"("曲线引用"=w772, "曲线索引"=1, "X"=w764, "Y"=w762) -> ()  [unwired: 10 in, 2 out]
                  }
                }
                n556 = local write "力特性正向去程"(w731) -> ()
                n557 = local write "吸收电流"(w734) -> ()
                n558 = local write "输入扭矩"(w732) -> ()
                n559 = local write "输出扭矩(大)"(w733) -> ()
                n560 = local write "T1+T2"(w735) -> ()
                n561 = local write "T1"(w737) -> ()
                n562 = local write "T2"(w736) -> ()
                "布尔" <- TRUE ("布尔")
              }
              frame 133 {
                n563 = local write "STEP"("等待" ("STEP")) -> ()
                n564 = call "设备状态.vi"("枚举"=enum16{"Read", "Write"}."Write", "Status_Write"=i16 134 ("设备状态")) -> ()  [unwired: 9 in, 1 out]
                n565 = disable-structure shown="禁用" {
                  frame Disabled {
                    n566 = global read "A180648.vi" "当前检测项"() -> (w778:T3)
                    n567 = case shown="\"力特性\"" w778 {
                      frame Default {
                      }
                      frame "力特性" {
                        n568 = call-poly "模式选择.vi"("Max Torque"=200.0, "Velocity"=sgl -1.0) -> ()  [unwired: 9 in, 1 out]
                      }
                    }
                  }
                  frame Enabled {
                  }
                }
              }
              frame 134 {
                n569 = control-ref of="电流特性试验"() -> (w785:refnum<vi>)
                n570 = local read "当前车速"() -> (w782:i32)
                n571 = global read "Global.vi" "传感器读数"() -> (w781:T18)
                n572 = control-ref of="力特性试验"() -> (w783:refnum<vi>)
                n573 = control-ref of="传感器特性试验"() -> (w784:refnum<vi>)
                n574 = local read "力特性正向回程"() -> (w786:bool)
                n575 = case shown="0, 默认" w782 {
                  selector: w782 -> [w808 _]
                  tunnel: w781 -> [w813 w829]
                  tunnel: w783 -> [w812 _]
                  tunnel: w784 -> [_ w827]
                  tunnel: w785 -> [w810 _]
                  tunnel: w786 -> [w799 w815]
                  tunnel: [FALSE FALSE] -> w787
                  tunnel: [w800 w819] -> w788
                  tunnel: [w802 _] -> w789
                  tunnel: [w801 _] -> w790
                  tunnel: [_ w818] -> w791
                  tunnel: [_ w817] -> w792
                  tunnel: [_ w816] -> w793
                  tunnel: 10 -> [w798 w814]
                  frame 0, Default {
                    n576 = Unbundle By Name(w813) -> ("输入扭矩"=w811:sgl, "输出扭矩(大)"=w797:sgl, "吸收电流"=w809:sgl)
                    n577 = Multiply(x=w808, y=4) -> (x*y=w805:i32)
                    n578 = Subtract(x=w797, y=sgl -0.2) -> (x-y=w795:sgl)
                    n579 = call-poly <userlib>:"MGI Running Average.vi"("Averaging Size"=w798, "Initialize? (F)"=w799, "Value"=w809) -> ("Average"=w801:sgl)  [unwired: 8 in]
                    n580 = call-poly <userlib>:"MGI Running Average.vi"("Averaging Size"=w798, "Initialize? (F)"=w799, "Value"=w811) -> ("Average"=w800:sgl)  [unwired: 8 in]
                    n581 = call-poly <userlib>:"MGI Running Average.vi"("Averaging Size"=w798, "Initialize? (F)"=w799, "Value"=w795) -> ("Average"=w802:sgl)  [unwired: 8 in]
                    n582 = Add(x=w805, y=1) -> (x+y=w804:i32)
                    n583 = call "曲线采集.vi"("曲线引用"=w810, "曲线索引"=w804, "X"=w800, "Y"=w801) -> ()  [unwired: 10 in, 2 out]
                    n584 = call "曲线采集.vi"("曲线引用"=w812, "曲线索引"=w804, "X"=w800, "Y"=w802) -> ()  [unwired: 10 in, 2 out]
                  }
                  frame 100 {
                    n585 = Unbundle By Name(w829) -> ("输入扭矩"=w828:sgl)
                    n586 = call "占空比.vi"() -> ("T1+T2"=w824:dbl, "T2"=w825:dbl, "T1"=w826:dbl)  [unwired: 9 in]
                    n587 = call-poly <userlib>:"MGI Running Average.vi"("Averaging Size"=w814, "Initialize? (F)"=w815, "Value"=w828) -> ("Average"=w819:sgl)  [unwired: 8 in]
                    n588 = call-poly <userlib>:"MGI Running Average.vi"("Averaging Size"=w814, "Initialize? (F)"=w815, "Value"=w824) -> ("Average"=w818:dbl)  [unwired: 8 in]
                    n589 = call-poly <userlib>:"MGI Running Average.vi"("Averaging Size"=w814, "Initialize? (F)"=w815, "Value"=w826) -> ("Average"=w816:dbl)  [unwired: 8 in]
                    n590 = call-poly <userlib>:"MGI Running Average.vi"("Averaging Size"=w814, "Initialize? (F)"=w815, "Value"=w825) -> ("Average"=w817:dbl)  [unwired: 8 in]
                    n591 = call "曲线采集.vi"("曲线引用"=w827, "曲线索引"=5, "X"=w819, "Y"=w818) -> ()  [unwired: 10 in, 2 out]
                    n592 = call "曲线采集.vi"("曲线引用"=w827, "曲线索引"=3, "X"=w819, "Y"=w816) -> ()  [unwired: 10 in, 2 out]
                    n593 = call "曲线采集.vi"("曲线引用"=w827, "曲线索引"=4, "X"=w819, "Y"=w817) -> ()  [unwired: 10 in, 2 out]
                  }
                }
                n594 = local write "力特性正向回程"(w787) -> ()
                n595 = local write "吸收电流"(w790) -> ()
                n596 = local write "输入扭矩"(w788) -> ()
                n597 = local write "输出扭矩(大)"(w789) -> ()
                n598 = local write "T1+T2"(w791) -> ()
                n599 = local write "T1"(w793) -> ()
                n600 = local write "T2"(w792) -> ()
              }
              frame 135 {
                n601 = call "设备状态.vi"("枚举"=enum16{"Read", "Write"}."Write", "Status_Write"=i16 136 ("设备状态")) -> ()  [unwired: 9 in, 1 out]
                n602 = local write "STEP"("等待" ("STEP")) -> ()
              }
              frame 136 {
                n603 = local read "力特性逆向去程"() -> (w838:bool)
                n604 = control-ref of="电流特性试验"() -> (w837:refnum<vi>)
                n605 = local read "当前车速"() -> (w834:i32)
                n606 = global read "Global.vi" "传感器读数"() -> (w833:T18)
                n607 = control-ref of="力特性试验"() -> (w835:refnum<vi>)
                n608 = control-ref of="传感器特性试验"() -> (w836:refnum<vi>)
                n609 = case shown="100" w834 {
                  selector: w834 -> [w860 _]
                  tunnel: w833 -> [w865 w881]
                  tunnel: w835 -> [w864 _]
                  tunnel: w836 -> [_ w879]
                  tunnel: w837 -> [w862 _]
                  tunnel: w838 -> [w851 w867]
                  tunnel: [FALSE FALSE] -> w839
                  tunnel: [w852 w871] -> w840
                  tunnel: [w854 _] -> w841
                  tunnel: [w853 _] -> w842
                  tunnel: [_ w870] -> w843
                  tunnel: [_ w869] -> w844
                  tunnel: [_ w868] -> w845
                  tunnel: 10 -> [w850 w866]
                  frame 0, Default {
                    n610 = Unbundle By Name(w865) -> ("输入扭矩"=w863:sgl, "输出扭矩(大)"=w849:sgl, "吸收电流"=w861:sgl)
                    n611 = Multiply(x=w860, y=4) -> (x*y=w857:i32)
                    n612 = Subtract(x=w849, y=sgl 0.0) -> (x-y=w848:sgl)
                    n613 = call-poly <userlib>:"MGI Running Average.vi"("Averaging Size"=w850, "Initialize? (F)"=w851, "Value"=w861) -> ("Average"=w853:sgl)  [unwired: 8 in]
                    n614 = call-poly <userlib>:"MGI Running Average.vi"("Averaging Size"=w850, "Initialize? (F)"=w851, "Value"=w863) -> ("Average"=w852:sgl)  [unwired: 8 in]
                    n615 = call-poly <userlib>:"MGI Running Average.vi"("Averaging Size"=w850, "Initialize? (F)"=w851, "Value"=w848) -> ("Average"=w854:sgl)  [unwired: 8 in]
                    n616 = Add(x=w857, y=2) -> (x+y=w856:i32)
                    n617 = call "曲线采集.vi"("曲线引用"=w862, "曲线索引"=w856, "X"=w852, "Y"=w853) -> ()  [unwired: 10 in, 2 out]
                    n618 = call "曲线采集.vi"("曲线引用"=w864, "曲线索引"=w856, "X"=w852, "Y"=w854) -> ()  [unwired: 10 in, 2 out]
                  }
                  frame 100 {
                    n619 = Unbundle By Name(w881) -> ("输入扭矩"=w880:sgl)
                    n620 = call "占空比.vi"() -> ("T1+T2"=w876:dbl, "T2"=w877:dbl, "T1"=w878:dbl)  [unwired: 9 in]
                    n621 = call-poly <userlib>:"MGI Running Average.vi"("Averaging Size"=w866, "Initialize? (F)"=w867, "Value"=w880) -> ("Average"=w871:sgl)  [unwired: 8 in]
                    n622 = call-poly <userlib>:"MGI Running Average.vi"("Averaging Size"=w866, "Initialize? (F)"=w867, "Value"=w876) -> ("Average"=w870:dbl)  [unwired: 8 in]
                    n623 = call-poly <userlib>:"MGI Running Average.vi"("Averaging Size"=w866, "Initialize? (F)"=w867, "Value"=w878) -> ("Average"=w868:dbl)  [unwired: 8 in]
                    n624 = call-poly <userlib>:"MGI Running Average.vi"("Averaging Size"=w866, "Initialize? (F)"=w867, "Value"=w877) -> ("Average"=w869:dbl)  [unwired: 8 in]
                    n625 = call "曲线采集.vi"("曲线引用"=w879, "曲线索引"=8, "X"=w871, "Y"=w870) -> ()  [unwired: 10 in, 2 out]
                    n626 = call "曲线采集.vi"("曲线引用"=w879, "曲线索引"=6, "X"=w871, "Y"=w868) -> ()  [unwired: 10 in, 2 out]
                    n627 = call "曲线采集.vi"("曲线引用"=w879, "曲线索引"=7, "X"=w871, "Y"=w869) -> ()  [unwired: 10 in, 2 out]
                  }
                }
                n628 = local write "力特性逆向去程"(w839) -> ()
                n629 = local write "吸收电流"(w842) -> ()
                n630 = local write "输入扭矩"(w840) -> ()
                n631 = local write "输出扭矩(大)"(w841) -> ()
                n632 = local write "T1+T2"(w843) -> ()
                n633 = local write "T1"(w845) -> ()
                n634 = local write "T2"(w844) -> ()
              }
              frame 137 {
                n635 = disable-structure shown="禁用" {
                  frame Disabled {
                    n636 = global read "A180648.vi" "当前检测项"() -> (w885:T3)
                    n637 = case shown="\"力特性\"" w885 {
                      frame Default {
                      }
                      frame "力特性" {
                        n638 = call-poly "模式选择.vi"("Max Torque"=200.0, "Velocity"=sgl 1.0) -> ()  [unwired: 9 in, 1 out]
                      }
                    }
                  }
                  frame Enabled {
                  }
                }
                n639 = call "设备状态.vi"("枚举"=enum16{"Read", "Write"}."Write", "Status_Write"=i16 138 ("设备状态")) -> ()  [unwired: 9 in, 1 out]
                n640 = local write "STEP"("等待" ("STEP")) -> ()
              }
              frame 138 {
                n641 = control-ref of="电流特性试验"() -> (w893:refnum<vi>)
                n642 = local read "当前车速"() -> (w890:i32)
                n643 = global read "Global.vi" "传感器读数"() -> (w889:T18)
                n644 = control-ref of="力特性试验"() -> (w891:refnum<vi>)
                n645 = control-ref of="传感器特性试验"() -> (w892:refnum<vi>)
                n646 = local read "力特性逆向回程"() -> (w894:bool)
                n647 = case shown="100" w890 {
                  selector: w890 -> [w915 _]
                  tunnel: w889 -> [w920 w936]
                  tunnel: w891 -> [w919 _]
                  tunnel: w892 -> [_ w934]
                  tunnel: w893 -> [w917 _]
                  tunnel: w894 -> [w906 w922]
                  tunnel: [FALSE FALSE] -> w895
                  tunnel: [w907 w926] -> w896
                  tunnel: [w909 _] -> w897
                  tunnel: [w908 _] -> w898
                  tunnel: [_ w925] -> w899
                  tunnel: [_ w924] -> w900
                  tunnel: [_ w923] -> w901
                  tunnel: 10 -> [w905 w921]
                  frame 0, Default {
                    n648 = Unbundle By Name(w920) -> ("输入扭矩"=w918:sgl, "输出扭矩(大)"=w904:sgl, "吸收电流"=w916:sgl)
                    n649 = Multiply(x=w915, y=4) -> (x*y=w912:i32)
                    n650 = Subtract(x=w904, y=sgl 0.0) -> (x-y=w902:sgl)
                    n651 = call-poly <userlib>:"MGI Running Average.vi"("Averaging Size"=w905, "Initialize? (F)"=w906, "Value"=w916) -> ("Average"=w908:sgl)  [unwired: 8 in]
                    n652 = call-poly <userlib>:"MGI Running Average.vi"("Averaging Size"=w905, "Initialize? (F)"=w906, "Value"=w902) -> ("Average"=w909:sgl)  [unwired: 8 in]
                    n653 = call-poly <userlib>:"MGI Running Average.vi"("Averaging Size"=w905, "Initialize? (F)"=w906, "Value"=w918) -> ("Average"=w907:sgl)  [unwired: 8 in]
                    n654 = Add(x=w912, y=3) -> (x+y=w911:i32)
                    n655 = call "曲线采集.vi"("曲线引用"=w917, "曲线索引"=w911, "X"=w907, "Y"=w908) -> ()  [unwired: 10 in, 2 out]
                    n656 = call "曲线采集.vi"("曲线引用"=w919, "曲线索引"=w911, "X"=w907, "Y"=w909) -> ()  [unwired: 10 in, 2 out]
                  }
                  frame 100 {
                    n657 = Unbundle By Name(w936) -> ("输入扭矩"=w935:sgl)
                    n658 = call "占空比.vi"() -> ("T1+T2"=w931:dbl, "T2"=w932:dbl, "T1"=w933:dbl)  [unwired: 9 in]
                    n659 = call-poly <userlib>:"MGI Running Average.vi"("Averaging Size"=w921, "Initialize? (F)"=w922, "Value"=w935) -> ("Average"=w926:sgl)  [unwired: 8 in]
                    n660 = call-poly <userlib>:"MGI Running Average.vi"("Averaging Size"=w921, "Initialize? (F)"=w922, "Value"=w931) -> ("Average"=w925:dbl)  [unwired: 8 in]
                    n661 = call-poly <userlib>:"MGI Running Average.vi"("Averaging Size"=w921, "Initialize? (F)"=w922, "Value"=w933) -> ("Average"=w923:dbl)  [unwired: 8 in]
                    n662 = call-poly <userlib>:"MGI Running Average.vi"("Averaging Size"=w921, "Initialize? (F)"=w922, "Value"=w932) -> ("Average"=w924:dbl)  [unwired: 8 in]
                    n663 = call "曲线采集.vi"("曲线引用"=w934, "曲线索引"=11, "X"=w926, "Y"=w925) -> ()  [unwired: 10 in, 2 out]
                    n664 = call "曲线采集.vi"("曲线引用"=w934, "曲线索引"=9, "X"=w926, "Y"=w923) -> ()  [unwired: 10 in, 2 out]
                    n665 = call "曲线采集.vi"("曲线引用"=w934, "曲线索引"=10, "X"=w926, "Y"=w924) -> ()  [unwired: 10 in, 2 out]
                  }
                }
                n666 = local write "力特性逆向回程"(w895) -> ()
                n667 = local write "吸收电流"(w898) -> ()
                n668 = local write "输入扭矩"(w896) -> ()
                n669 = local write "输出扭矩(大)"(w897) -> ()
                n670 = local write "T1+T2"(w899) -> ()
                n671 = local write "T1"(w901) -> ()
                n672 = local write "T2"(w900) -> ()
              }
              frame 139 {
                n673 = local read "布尔"() -> (w937:bool)
                n674 = case shown="真" w937 {
                  frame False {
                  }
                  frame True {
                    n675 = global read "A180648.vi" "车速"() -> (w941:sgl[])
                    n676 = local write "布尔"(FALSE ("布尔")) -> ()
                    n677 = Array Size(array=w941) -> (size(s)=w943:i32)
                    n678 = local read "当前车速"() -> (w940:i32)
                    n679 = Decrement(x=w943) -> (x-1=w939:i32)
                    n680 = Greater Or Equal?(x=w940, y=w939) -> (x >= y?=w942:bool)
                    n681 = case shown="假" w942 {
                      frame False {
                        n682 = stacked-sequence {
                          frame #0 {
                            n683 = local read "当前车速"() -> (w945:i32)
                            n684 = Increment(x=w945) -> (x+1=w944:i32)
                            n685 = local write "当前车速"(w944) -> ()
                          }
                          frame #1 {
                            w953 = u16 2 items=["byte", "word", "Dword"] ("数据类型")
                            w956 = u8 132 items=["I/O (P)"=128, "Input (I)"=129, "Output (Q)"=130, "Bit Memory (M)"=131, "Data (DB)"=132, "Instance Data (DI)"=133, "Local Data (L)"=134, "Predecessor Local Data (VL)"=135] ("寄存器类型")
                            n686 = local read "当前车速"() -> (w949:i32)
                            n687 = global read "A180648.vi" "车速"() -> (w950:sgl[])
                            n688 = Index Array(array=w950, index=w949) -> (element=w946:sgl)
                            n689 = Type Cast(type=u32 0, x=w946) -> (*(type *) &x=w951:u32)
                            n690 = Round Toward +Infinity(x=w946) -> (ceil(x): smallest int >= x=w948:sgl)
                            n691 = call "Write_Data.vi"("DB #"=u16 7, "寄存器类型"=w956, "写入数据"=w951, "数据类型"=w953, "写入地址"=u32 160) -> ()  [unwired: 4 in, 3 out]
                            n692 = To Unsigned Word Integer(number=w948) -> (unsigned 16bit integer=w947:u16)
                            n693 = global write "A180648.vi" "当前车速"(w947) -> ()
                          }
                          frame #2 {
                            n694 = call "设备状态.vi"("枚举"=enum16{"Read", "Write"}."Write", "Status_Write"=i16 132 ("设备状态")) -> ()  [unwired: 9 in, 1 out]
                          }
                          frame #3 {
                            n695 = disable-structure shown="禁用" {
                              frame Disabled {
                                n696 = global read "A180648.vi" "当前检测项"() -> (w959:T3)
                                n697 = case shown="\"力特性\"" w959 {
                                frame Default {
                                }
                                frame "力特性" {
                                n698 = call-poly "模式选择.vi"("Max Torque"=200.0, "Velocity"=sgl -1.0) -> ()  [unwired: 9 in, 1 out]
                                }
                                }
                              }
                              frame Enabled {
                              }
                            }
                          }
                          frame #4 {
                            w962 = TRUE
                            n699 = local write "力特性逆向回程"(w962) -> ()
                            n700 = local write "力特性正向去程"(w962) -> ()
                            n701 = local write "力特性逆向去程"(w962) -> ()
                            n702 = local write "力特性正向回程"(w962) -> ()
                          }
                        }
                      }
                      frame True {
                        n703 = local write "STEP"("判定" ("STEP")) -> ()
                        n704 = call-poly "模式选择.vi"("Max Torque"=200.0, "Velocity"=sgl 0.0) -> ()  [unwired: 9 in, 1 out]
                      }
                    }
                  }
                }
              }
              frame 142 {
                n705 = stacked-sequence {
                  frame #0 {
                    n706 = global read "Global.vi" "输出占空比"() -> (w969:refnum<vi>)
                    n707 = call "设备状态.vi"("枚举"=enum16{"Read", "Write"}."Write", "Status_Write"=i16 143) -> ()  [unwired: 9 in, 1 out]
                    n708 = property class="Num"(reference=w969, "Val(Sgnl)"=52.0) -> ()  [unwired: 1 in, 2 out]
                  }
                  frame #1 {
                    n709 = Wait (ms)(milliseconds to wait=u32 2000 ("等待时间（毫秒）")) -> ()  [unwired: 1 out]
                  }
                }
              }
              frame 143 {
                n710 = stacked-sequence {
                  frame #0 {
                    n711 = control-ref of="振动1NVH-FFT"() -> (w975:refnum<vi>)
                    n712 = control-ref of="振动2NHV-FFT"() -> (w974:refnum<vi>)
                    n713 = call "振动检测.vi"("振动一"=w975, "通道输入"=tag "cDaq1Mod1/ai1:2" ("DAQmx物理通道"), "振动二"=w974, "重置"=FALSE) -> ("spectrum info"=w973:T19[])  [unwired: 10 in, 1 out]
                    n714 = global write "Global.vi" "spectrum info"(w973) -> ()
                  }
                  frame #1 {
                    n715 = global read "Global.vi" "输出占空比"() -> (w979:refnum<vi>)
                    n716 = call "设备状态.vi"("枚举"=enum16{"Read", "Write"}."Write", "Status_Write"=i16 144) -> ()  [unwired: 9 in, 1 out]
                    n717 = property class="Num"(reference=w979, "Val(Sgnl)"=48.0) -> ()  [unwired: 1 in, 2 out]
                  }
                  frame #2 {
                    n718 = Wait (ms)(milliseconds to wait=u32 2000 ("等待时间（毫秒）")) -> ()  [unwired: 1 out]
                  }
                }
              }
              frame 144 {
                n719 = stacked-sequence {
                  frame #0 {
                    n720 = control-ref of="振动1NVH-FFT"() -> (w985:refnum<vi>)
                    n721 = control-ref of="振动2NHV-FFT"() -> (w984:refnum<vi>)
                    n722 = call "振动检测.vi"("振动一"=w985, "通道输入"=tag "cDaq1Mod1/ai1:2" ("DAQmx物理通道"), "振动二"=w984, "重置"=FALSE) -> ("spectrum info"=w983:T19[])  [unwired: 10 in, 1 out]
                    n723 = global write "Global.vi" "spectrum info"(w983) -> ()
                  }
                  frame #1 {
                    n724 = call "设备状态.vi"("枚举"=enum16{"Read", "Write"}."Write", "Status_Write"=i16 145) -> ()  [unwired: 9 in, 1 out]
                  }
                }
              }
              frame 146 {
                n725 = local write "STEP"("判定" ("STEP")) -> ()
              }
              frame 152 {
                n726 = global read "A180648.vi" "当前检测项"() -> (w989:T3)
                n727 = case shown="\"磨合\"" w989 {
                  frame "逆向空载", Default {
                    n728 = global read "A180648.vi" "逆向空载试验参数"() -> (w995:T25)
                    n729 = Unbundle By Name(w995) -> ("启用助力"=w992:dbl, "试验速度"=w994:dbl)
                    n730 = case shown="0, 默认" w992 {
                      frame 0, Default {
                        n731 = call "设备状态.vi"("枚举"=enum16{"Read", "Write"}."Write", "Status_Write"=i16 154 ("设备状态")) -> ()  [unwired: 9 in, 1 out]
                      }
                      frame 1 {
                        n732 = call "设备状态.vi"("枚举"=enum16{"Read", "Write"}."Write", "Status_Write"=i16 155 ("设备状态")) -> ()  [unwired: 9 in, 1 out]
                      }
                    }
                    n733 = call-poly "模式选择.vi"("Reset Count"=TRUE, "Max Torque"=50.0, "Velocity"=w994) -> ()  [unwired: 8 in, 1 out]
                  }
                  frame "磨合" {
                    n734 = global read "A180648.vi" "磨合试验参数"() -> (w1004:T25)
                    n735 = Unbundle By Name(w1004) -> ("启用助力"=w1002:dbl, "试验速度"=w1003:dbl)
                    n736 = case shown="0, 默认" w1002 {
                      frame 0, Default {
                        n737 = call "设备状态.vi"("枚举"=enum16{"Read", "Write"}."Write", "Status_Write"=i16 154 ("设备状态")) -> ()  [unwired: 9 in, 1 out]
                      }
                      frame 1 {
                        n738 = call "设备状态.vi"("枚举"=enum16{"Read", "Write"}."Write", "Status_Write"=i16 155 ("设备状态")) -> ()  [unwired: 9 in, 1 out]
                      }
                    }
                    n739 = call-poly "模式选择.vi"("Reset Count"=TRUE, "Max Torque"=50.0, "Velocity"=w1003) -> ()  [unwired: 8 in, 1 out]
                  }
                }
                n740 = local write "STEP"("等待" ("STEP")) -> ()
              }
              frame 154, 155 {
                n741 = global read "A180648.vi" "当前检测项"() -> (w1009:T3)
                n742 = case shown="\"磨合\"" w1009 {
                  frame "逆向空载", Default {
                    n743 = global read "System_Conf.vi" "system"() -> (w1012:T8)
                    n744 = Unbundle By Name(w1012) -> ("逆向空载滤波"=w1011:bool, "逆向空载扭矩系数"=w1010:dbl)
                    n745 = call "传感器数据.vi"() -> ("传感器读数"=w1026:T18)  [unwired: 11 in]
                    n746 = local read "逆向空载正向初始化"() -> (w1027:bool)
                    n747 = Unbundle By Name(w1026) -> ("输出扭矩(小)"=w1013:sgl)
                    n748 = global read "A180648.vi" "逆向空载试验参数"() -> (w1025:T25)
                    n749 = Multiply(x=w1013, y=w1010) -> (x*y=w1014:dbl)
                    n750 = call "GetActualPosition.vi"() -> ("Axis_ActualPosition(°)"=w1017:dbl)  [unwired: 11 in]
                    n751 = case shown="真" w1011 {
                      tunnel: w1017 -> [w1029 w1035]
                      tunnel: [w1029 w1034] -> w1016
                      tunnel: [w1028 w1033] -> w1015
                      tunnel: w1014 -> [w1028 w1031]
                      tunnel: w1027 -> [_ w1030]
                      frame False {
                      }
                      frame True {
                        w1032 = 10 ("Averaging Size")
                        n752 = call-poly <userlib>:"MGI Running Average.vi"("Averaging Size"=w1032, "Initialize? (F)"=w1030, "Value"=w1035) -> ("Average"=w1034:dbl)  [unwired: 8 in]
                        n753 = call-poly <userlib>:"MGI Running Average.vi"("Averaging Size"=w1032, "Initialize? (F)"=w1030, "Value"=w1031) -> ("Average"=w1033:dbl)  [unwired: 8 in]
                      }
                    }
                    n754 = Unbundle By Name(w1025) -> ("试验速度"=w1018:dbl, "试验角度"=w1024:dbl, "保护扭矩"=w1023:dbl, "启用助力"=w1019:dbl)
                    n755 = Less Or Equal?(x=w1016, y=w1024) -> (x <= y?=w1021:bool)
                    n756 = Less Or Equal?(x=w1015, y=w1023) -> (x <= y?=w1020:bool)
                    n757 = And(x=w1021, y=w1020) -> (x .and. y?=w1022:bool)
                    n758 = case shown="假" w1022 {
                      tunnel: w1016 -> [_ w1051]
                      tunnel: w1015 -> [_ w1050]
                      tunnel: w1019 -> [w1037 _]
                      tunnel: w1018 -> [w1036 _]
                      frame False {
                        n759 = stacked-sequence {
                          tunnel: w1037 -> [_ w1038 _ _]
                          tunnel: w1036 -> [_ _ w1046 _]
                          frame #0 {
                            n760 = call-poly "模式选择.vi"() -> ()  [unwired: 11 in, 1 out]
                          }
                          frame #1 {
                            n761 = case shown="0, 默认" w1038 {
                              frame 0, Default {
                                n762 = call "设备状态.vi"("枚举"=enum16{"Read", "Write"}."Write", "Status_Write"=i16 156 ("设备状态")) -> ()  [unwired: 9 in, 1 out]
                              }
                              frame 1 {
                                n763 = call "设备状态.vi"("枚举"=enum16{"Read", "Write"}."Write", "Status_Write"=i16 157 ("设备状态")) -> ()  [unwired: 9 in, 1 out]
                              }
                            }
                          }
                          frame #2 {
                            n764 = Negate(x=w1046) -> (-x=w1045:dbl)
                            n765 = call-poly "模式选择.vi"("Reset Count"=FALSE, "Max Torque"=50.0, "Velocity"=w1045) -> ()  [unwired: 8 in, 1 out]
                          }
                          frame #3 {
                            n766 = local write "STEP"("等待" ("STEP")) -> ()
                          }
                        }
                      }
                      frame True {
                        n767 = control-ref of="逆向空载试验"() -> (w1053:refnum<vi>)
                        n768 = call "曲线采集.vi"("曲线引用"=w1053, "曲线索引"=0, "X"=w1051, "Y"=w1050) -> ("错误输出"=w1049:errorcluster)  [unwired: 10 in, 1 out]
                        n769 = Unbundle By Name(w1049) -> ("status"=w1048:bool)
                        n770 = local write "逆向空载正向初始化"(w1048) -> ()
                      }
                    }
                  }
                  frame "磨合" {
                    w1054 = 10 ("Averaging Size")
                    n771 = local read "磨合正向初始化"() -> (w1068:bool)
                    n772 = call "传感器数据.vi"() -> ("传感器读数"=w1067:T18)  [unwired: 11 in]
                    n773 = Unbundle By Name(w1067) -> ("输出扭矩(大)"=w1055:sgl)
                    n774 = global read "A180648.vi" "磨合试验参数"() -> (w1066:T25)
                    n775 = call "GetActualPosition.vi"() -> ("Axis_ActualPosition(°)"=w1058:dbl)  [unwired: 11 in]
                    n776 = Unbundle By Name(w1066) -> ("试验速度"=w1059:dbl, "试验角度"=w1065:dbl, "保护扭矩"=w1064:dbl, "启用助力"=w1060:dbl)
                    n777 = call-poly <userlib>:"MGI Running Average.vi"("Averaging Size"=w1054, "Initialize? (F)"=w1068, "Value"=w1058) -> ("Average"=w1057:dbl)  [unwired: 8 in]
                    n778 = call-poly <userlib>:"MGI Running Average.vi"("Averaging Size"=w1054, "Initialize? (F)"=w1068, "Value"=w1055) -> ("Average"=w1056:sgl)  [unwired: 8 in]
                    n779 = Less Or Equal?(x=w1057, y=w1065) -> (x <= y?=w1062:bool)
                    n780 = Less Or Equal?(x=w1056, y=w1064) -> (x <= y?=w1061:bool)
                    n781 = And(x=w1062, y=w1061) -> (x .and. y?=w1063:bool)
                    n782 = case shown="真" w1063 {
                      tunnel: w1057 -> [_ w1085]
                      tunnel: w1056 -> [_ w1084]
                      tunnel: w1060 -> [w1070 _]
                      tunnel: w1059 -> [w1069 _]
                      frame False {
                        n783 = stacked-sequence {
                          tunnel: w1070 -> [_ w1071 _ _]
                          tunnel: w1069 -> [_ _ w1079 _]
                          frame #0 {
                            n784 = call-poly "模式选择.vi"() -> ()  [unwired: 11 in, 1 out]
                          }
                          frame #1 {
                            n785 = case shown="0, 默认" w1071 {
                              frame 0, Default {
                                n786 = call "设备状态.vi"("枚举"=enum16{"Read", "Write"}."Write", "Status_Write"=i16 156 ("设备状态")) -> ()  [unwired: 9 in, 1 out]
                              }
                              frame 1 {
                                n787 = call "设备状态.vi"("枚举"=enum16{"Read", "Write"}."Write", "Status_Write"=i16 157 ("设备状态")) -> ()  [unwired: 9 in, 1 out]
                              }
                            }
                          }
                          frame #2 {
                            n788 = Negate(x=w1079) -> (-x=w1078:dbl)
                            n789 = call-poly "模式选择.vi"("Reset Count"=FALSE, "Max Torque"=50.0, "Velocity"=w1078) -> ()  [unwired: 8 in, 1 out]
                          }
                          frame #3 {
                            n790 = local write "STEP"("等待" ("STEP")) -> ()
                          }
                        }
                      }
                      frame True {
                        n791 = control-ref of="磨合"() -> (w1081:refnum<vi>)
                        n792 = call "曲线采集.vi"("曲线引用"=w1081, "曲线索引"=0, "X"=w1085, "Y"=w1084) -> ("错误输出"=w1083:errorcluster)  [unwired: 10 in, 1 out]
                        n793 = Unbundle By Name(w1083) -> ("status"=w1082:bool)
                        n794 = local write "磨合正向初始化"(w1082) -> ()
                      }
                    }
                  }
                }
              }
              frame 156, 157 {
                n795 = global read "A180648.vi" "当前检测项"() -> (w1087:T3)
                n796 = case shown="\"逆向空载\", 默认" w1087 {
                  frame "逆向空载", Default {
                    n797 = global read "System_Conf.vi" "system"() -> (w1090:T8)
                    n798 = call "传感器数据.vi"() -> ("传感器读数"=w1093:T18)  [unwired: 11 in]
                    n799 = Unbundle By Name(w1090) -> ("逆向空载滤波"=w1089:bool, "逆向空载扭矩系数"=w1088:dbl)
                    n800 = Unbundle By Name(w1093) -> ("输出扭矩(小)"=w1092:sgl)
                    n801 = local read "逆向空载逆向初始化"() -> (w1094:bool)
                    n802 = global read "A180648.vi" "逆向空载试验参数"() -> (w1103:T25)
                    n803 = call "GetActualPosition.vi"() -> ("Axis_ActualPosition(°)"=w1096:dbl)  [unwired: 11 in]
                    n804 = Multiply(x=w1092, y=w1088) -> (x*y=w1091:dbl)
                    n805 = case shown="真" w1089 {
                      tunnel: w1091 -> [w1104 w1111]
                      tunnel: w1094 -> [_ w1110]
                      tunnel: [w1105 w1109] -> w1095
                      tunnel: w1096 -> [w1105 w1108]
                      tunnel: [w1104 w1107] -> w1097
                      frame False {
                      }
                      frame True {
                        w1106 = 10 ("Averaging Size")
                        n806 = call-poly <userlib>:"MGI Running Average.vi"("Averaging Size"=w1106, "Initialize? (F)"=w1110, "Value"=w1108) -> ("Average"=w1109:dbl)  [unwired: 8 in]
                        n807 = call-poly <userlib>:"MGI Running Average.vi"("Averaging Size"=w1106, "Initialize? (F)"=w1110, "Value"=w1111) -> ("Average"=w1107:dbl)  [unwired: 8 in]
                      }
                    }
                    n808 = Unbundle By Name(w1103) -> ("保护扭矩"=w1102:dbl)
                    n809 = Negate(x=w1102) -> (-x=w1098:dbl)
                    n810 = Greater Or Equal To 0?(x=w1095) -> (x >= 0?=w1100:bool)
                    n811 = Greater Or Equal?(x=w1097, y=w1098) -> (x >= y?=w1099:bool)
                    n812 = And(x=w1100, y=w1099) -> (x .and. y?=w1101:bool)
                    n813 = case shown="真" w1101 {
                      tunnel: w1095 -> [_ w1116]
                      tunnel: w1097 -> [_ w1115]
                      frame False {
                        n814 = stacked-sequence {
                          frame #0 {
                            n815 = call-poly "模式选择.vi"() -> ()  [unwired: 11 in, 1 out]
                          }
                          frame #1 {
                            n816 = local write "STEP"("判定" ("STEP")) -> ()
                          }
                        }
                      }
                      frame True {
                        n817 = control-ref of="逆向空载试验"() -> (w1118:refnum<vi>)
                        n818 = call "曲线采集.vi"("曲线引用"=w1118, "曲线索引"=1, "X"=w1116, "Y"=w1115) -> ("错误输出"=w1114:errorcluster)  [unwired: 10 in, 1 out]
                        n819 = Unbundle By Name(w1114) -> ("status"=w1113:bool)
                        n820 = local write "逆向空载逆向初始化"(w1113) -> ()
                      }
                    }
                  }
                  frame "磨合" {
                    w1120 = 10 ("Averaging Size")
                    n821 = local read "磨合逆向初始化"() -> (w1122:bool)
                    n822 = call "传感器数据.vi"() -> ("传感器读数"=w1121:T18)  [unwired: 11 in]
                    n823 = global read "A180648.vi" "磨合试验参数"() -> (w1131:T25)
                    n824 = call "GetActualPosition.vi"() -> ("Axis_ActualPosition(°)"=w1124:dbl)  [unwired: 11 in]
                    n825 = Unbundle By Name(w1121) -> ("输出扭矩(大)"=w1119:sgl)
                    n826 = Unbundle By Name(w1131) -> ("保护扭矩"=w1130:dbl)
                    n827 = call-poly <userlib>:"MGI Running Average.vi"("Averaging Size"=w1120, "Initialize? (F)"=w1122, "Value"=w1124) -> ("Average"=w1123:dbl)  [unwired: 8 in]
                    n828 = call-poly <userlib>:"MGI Running Average.vi"("Averaging Size"=w1120, "Initialize? (F)"=w1122, "Value"=w1119) -> ("Average"=w1125:sgl)  [unwired: 8 in]
                    n829 = Negate(x=w1130) -> (-x=w1126:dbl)
                    n830 = Greater Or Equal To 0?(x=w1123) -> (x >= 0?=w1128:bool)
                    n831 = Greater Or Equal?(x=w1125, y=w1126) -> (x >= y?=w1127:bool)
                    n832 = And(x=w1128, y=w1127) -> (x .and. y?=w1129:bool)
                    n833 = case shown="假" w1129 {
                      tunnel: w1123 -> [_ w1137]
                      tunnel: w1125 -> [_ w1136]
                      frame False {
                        n834 = stacked-sequence {
                          frame #0 {
                            n835 = call-poly "模式选择.vi"() -> ()  [unwired: 11 in, 1 out]
                          }
                          frame #1 {
                            n836 = local write "STEP"("判定" ("STEP")) -> ()
                          }
                        }
                      }
                      frame True {
                        n837 = control-ref of="磨合"() -> (w1133:refnum<vi>)
                        n838 = call "曲线采集.vi"("曲线引用"=w1133, "曲线索引"=1, "X"=w1137, "Y"=w1136) -> ("错误输出"=w1135:errorcluster)  [unwired: 10 in, 1 out]
                        n839 = Unbundle By Name(w1135) -> ("status"=w1134:bool)
                        n840 = local write "磨合逆向初始化"(w1134) -> ()
                      }
                    }
                  }
                }
              }
              frame 999 {
                n841 = call "浮动通知.vi"("通知内容"="请启动！" ("Status")) -> ()  [unwired: 11 in]
              }
              frame 1000 {
                n842 = local write "STEP"("初始化" ("STEP")) -> ()
              }
              frame 1024 {
                n843 = call "停止发送CAN.vi"() -> ()  [unwired: 11 in, 1 out]
                n844 = local write "STEP"("退出自动" ("STEP")) -> ()
              }
            }
          }
          frame "合格判定" {
            n845 = Wait (ms)(milliseconds to wait=u32 100 ("等待时间（毫秒）")) -> ()  [unwired: 1 out]
            n846 = local write "STEP"("等待" ("STEP")) -> ()
          }
          frame "报表" {
            n847 = stacked-sequence {
              seq-local: [_ w1149 _ _] -> [_ _ w1153 _]
              frame #0 {
                n848 = global write "Global.vi" "计时开始"(FALSE ("计时开始")) -> ()
              }
              frame #1 {
                n849 = global read "Global.vi" "产品编号"() -> (w1146:string)
                n850 = call <vilib>:"Space Constant.vi"() -> ("String"=w1148:string)
                n851 = call "时间秒.vi"() -> ("结果字符串"=w1147:string)  [unwired: 11 in]
                n852 = Concatenate Strings(w1146, w1148, w1147) -> (w1145:string)
                n853 = call "Report.vi"("文件重命名"=TRUE, "文件名称"=w1145, "检测结果"="判定结果") -> ("PRODUCT_VAULE"=w1149:string)  [unwired: 7 in, 1 out]
              }
              frame #2 {
                n854 = global read "Global.vi" "联机模式"() -> (w1152:enum16{"单机", "追溯"})
                n855 = case shown="\"追溯\"" w1152 {
                  tunnel: w1153 -> [_ w1154]
                  frame "单机", Default {
                  }
                  frame "追溯" {
                    n856 = global read "Global.vi" "Result"() -> (w1156:refnum<vi>)
                    n857 = property class="Tbl"(reference=w1156) -> (reference out=w1161:refnum<vi>, error out=w1158:errorcluster, "Row Headers[]"=w1159:string[])  [unwired: 1 in]
                    n858 = property class="Tbl"(reference=w1161, error in=w1158) -> (error out=w1157:errorcluster, "Value"=w1160:string[][])  [unwired: 1 out]
                    n859 = for {
                      tunnel: w1160 -> [w1168] mode=indexing
                      tunnel: w1159 -> [w1169] mode=indexing
                      tunnel: [w1166] -> w1155 mode=indexing if=w1167
                      shift-right: [w1165] -> _
                      shift-left: w1157 -> [w1165]
                      n860 = Build Array (concatenate)(w1169, w1168) -> (w1166:string[])
                      n861 = Index Array(array=w1168) -> (element=w1170:string)  [unwired: 1 in]
                      n862 = case shown="\"\"" w1170 {
                        tunnel: [TRUE FALSE] -> w1167
                        frame Default {
                        }
                        frame "" {
                        }
                      }
                    }
                    n863 = global read "追溯Global.vi" "DEVICE_ID"() -> (w1163:string)
                    n864 = global read "追溯Global.vi" "CODE_ID"() -> (w1164:string)
                    n865 = global read "追溯Global.vi" "USER_ID"() -> (w1162:string)
                    n866 = call "UPTEST.vi"("Result"=w1155, "CODE_ID"=w1164, "DEVICE_ID"=w1163) -> ()  [unwired: 6 in, 1 out]
                    n867 = call "UPRESULT.vi"("DEVICE_ID"=w1163, "USER_ID"=w1162, "CODE_ID"=w1164, "RESULT_VALUE"=w1154) -> ()  [unwired: 11 in, 1 out]
                  }
                }
              }
              frame #3 {
                n868 = local write "STEP"("进入自动" ("STEP")) -> ()
              }
            }
          }
        }
        n869 = global read "Global.vi" "程序关闭"() -> (w30:bool)
      }
      n870 = while {
        shift-right: [w1174] -> w27
        shift-left: w28 -> [w1175]
        stop <- w1176 stop-if-true
        n871 = event shown="[6] \"电流特性试验\", \"传感器特性试验\", \"力特性试验\", \"振动1NVH-FFT\", \"空载试验\", \"功能试验\", \"逆向空载试验\", \"磨合\": 鼠标进入;  \"电流特性试验\", \"传感器特性试验\", \"力特性试验\", \"振动1NVH-FFT\", \"空载试验\", \"功能试验\", \"逆向空载试验\", \"磨合\": 鼠标离开;  \"电流特性试验\", \"传感器特性试验\", \"力特性试验\", \"振动1NVH-FFT\", \"空载试验\", \"功能试验\", \"逆向空载试验\": 游标移动;  \"磨合\": 鼠标移动" {
          selector: w1175 -> [_ _ _ _ _ _ _ _]
          dyn-events: [_ _ _ _ _ _ _ _] -> w1174
          timeout: 200 -> [_ _ _ _ _ _ _ _]
          event Timeout {
            n872 = event-data() -> ()  [unwired: 1 in, 3 out]
            n873 = call "Obtain Broadcast Events for Registration.vi"() -> ("Already running?"=w1178:bool)  [unwired: 9 in, 2 out]
            n874 = case shown="真" w1178 {
              frame False {
                n875 = local write "STEP"("手动" ("STEP")) -> ()
              }
              frame True {
                n876 = call "错误代码.vi"() -> ("Status_Read"=w1180:u32)  [unwired: 11 in]
                n877 = feedback #1() -> (w1190:u32)  [unwired: 1 in]
                n878 = feedback-in #1(w1180) -> ()
                n879 = case shown="0" w1180 {
                  frame 0 {
                    n880 = global read "Global.vi" "报警图标"() -> (w1191:refnum<vi>)
                    n881 = property class="Bool"(reference=w1191, "Visible"=FALSE ("可见")) -> ()  [unwired: 1 in, 2 out]
                  }
                  frame 1, Default {
                    n882 = global read "Global.vi" "报警图标"() -> (w1194:refnum<vi>)
                    n883 = property class="Bool"(reference=w1194, "Visible"=TRUE ("可见")) -> ()  [unwired: 1 in, 2 out]
                  }
                }
                n884 = Greater Or Equal?(x=w1180, y=i16 5000) -> (x >= y?=w1188:bool)
                n885 = Less?(x=w1180, y=i16 5200) -> (x < y?=w1189:bool)
                n886 = Equal?(x=w1180, y=w1190) -> (x = y?=w1187:bool)
                n887 = global read "Global.vi" "报警图标"() -> (w1182:refnum<vi>)
                n888 = And(x=w1188, y=w1189) -> (x .and. y?=w1181:bool)
                n889 = property class="Bool"(reference=w1182, "Value"=w1181) -> ()  [unwired: 1 in, 2 out]
                n890 = Bundle By Name(cluster=errorcluster {"status"=FALSE, "code"=0, "source"=""} ("错误常量"), "status"=w1181, "code"=w1180) -> (w1186:errorcluster)
                n891 = case shown="假" w1187 {
                  tunnel: w1186 -> [w1195 _]
                  frame False {
                    n892 = call "报警处理.vi"("错误常量"=w1195) -> ()  [unwired: 9 in, 2 out]
                  }
                  frame True {
                  }
                }
              }
            }
          }
          event User Event {
            n893 = event-data() -> ("试验项"=w1196:T1)  [unwired: 1 in]
            "试验项目" <- w1196
            n894 = disable-structure shown="禁用" {
              disable-tunnel: w1196 -> [w1197 _]
              frame Disabled {
                n895 = global read "A180648.vi" "检测结果"() -> (w1200:string[][][])
                n896 = global read "Global.vi" "Result"() -> (w1198:refnum<vi>)
                n897 = Index Array(array=w1200, index (dim 0)=w1197) -> (element=w1199:string[][])  [unwired: 2 in]
                n898 = property class="Tbl"(reference=w1198, "Value"=w1199) -> ()  [unwired: 1 in, 2 out]
              }
              frame Enabled {
              }
            }
          }
          event "试验项目": Value Change {
            n899 = event-data() -> ("NewVal"=w1201:T1)  [unwired: 1 in]
            n900 = disable-structure shown="禁用" {
              disable-tunnel: w1201 -> [w1205 _]
              frame Disabled {
                n901 = global read "A180648.vi" "检测结果"() -> (w1204:string[][][])
                n902 = global read "Global.vi" "Result"() -> (w1202:refnum<vi>)
                n903 = Index Array(array=w1204, index (dim 0)=w1205) -> (element=w1203:string[][])  [unwired: 2 in]
                n904 = property class="Tbl"(reference=w1202, "Value"=w1203) -> ()  [unwired: 1 in, 2 out]
              }
              frame Enabled {
              }
            }
          }
          event "电流特性试验", "传感器特性试验", "力特性试验", "空载试验", "功能试验", "逆向空载试验", "磨合": Scale Range Change {
            n905 = event-data() -> ("CtlRef"=w1207:refnum<vi>)  [unwired: 1 in, 4 out]
            n906 = global read "Global.vi" "产品型号"() -> (w1206:string)
            n907 = call "XY_conf.vi"("方式"=enum16{"写入", "读取"}."写入", "产品"=w1206, "XY图引用"=w1207) -> ()  [unwired: 4 in, 1 out]
          }
          event User Event {
            n908 = event-data() -> ("产品"=w1209:string)  [unwired: 1 in]
            n909 = control-ref of="传感器特性试验"() -> (w1214:refnum<vi>)
            n910 = control-ref of="逆向空载试验"() -> (w1216:refnum<vi>)
            n911 = control-ref of="电流特性试验"() -> (w1215:refnum<vi>)
            n912 = control-ref of="力特性试验"() -> (w1213:refnum<vi>)
            n913 = control-ref of="功能试验"() -> (w1212:refnum<vi>)
            n914 = control-ref of="空载试验"() -> (w1211:refnum<vi>)
            n915 = Build Array(w1216, w1212, w1211, w1215, w1214, w1213) -> (w1210:refnum<vi>[])
            n916 = for {
              tunnel: w1210 -> [w1218] mode=indexing
              tunnel: w1209 -> [w1217]
              n917 = call "XY_conf.vi"("方式"=enum16{"写入", "读取"}."读取", "产品"=w1217, "XY图引用"=w1218) -> ()  [unwired: 4 in, 1 out]
            }
          }
          event Panel Close {
            n918 = event-data() -> ()  [unwired: 1 in, 4 out]
            n919 = global write "Global.vi" "程序关闭"(TRUE ("程序关闭")) -> ()
          }
          event "电流特性试验", "传感器特性试验", "力特性试验", "振动1NVH-FFT", "空载试验", "功能试验", "逆向空载试验", "磨合": Mouse Enter; "电流特性试验", "传感器特性试验", "力特性试验", "振动1NVH-FFT", "空载试验", "功能试验", "逆向空载试验", "磨合": Mouse Leave; "电流特性试验", "传感器特性试验", "力特性试验", "振动1NVH-FFT", "空载试验", "功能试验", "逆向空载试验": Cursor Move; "磨合": Mouse Move {
            n920 = event-data() -> ("CtlRef"=w1223:refnum<vi>, "Type"=w1221:T26)  [unwired: 1 in]
            n921 = call "CursorShow.vi"("nameShow"=TRUE, "Type"=w1221, "Graph"=w1223) -> ()  [unwired: 7 in, 2 out]
          }
          event "电流特性试验", "传感器特性试验", "力特性试验", "振动1NVH-FFT", "空载试验", "功能试验", "逆向空载试验", "磨合": Mouse Down {
            n922 = event-data() -> ("CtlRef"=w1228:refnum<vi>, "Coords"=w1227:T27, "Type"=w1225:T26)  [unwired: 1 in]
            n923 = invoke class="WFGraph" method="Map Coords To XY"(reference=w1228, "Coords"=w1227) -> (reference out=w1226:refnum<vi>, "XY"=w1224:cluster{"X":dbl, "Y":dbl})  [unwired: 5 in, 5 out]
            n924 = call "CursorShow.vi"("游标.游标位置"=w1224, "Type"=w1225, "Graph"=w1226) -> ()  [unwired: 7 in, 2 out]
          }
        }
        n925 = global read "Global.vi" "程序关闭"() -> (w1176:bool)
      }
    }
  }
  n926 = Unregister For Events(event registration refnum=w3) -> ()  [unwired: 1 in, 1 out]
